vi "RANGE Gas Meters.vi"() -> ()   [LabVIEW 2016]
uses:
  Type Definitions/RANGE DAQ Data Four Meters.ctl
  Type Definitions/RANGE DAQ Data.ctl
  Drivers/Omega FMA-1600A Series Gas Flow Meter/Type Definitions/FMA1600A Gas Type.ctl
  Drivers/Omega FMA-1600A Series Gas Flow Meter/Type Definitions/FMA1600A Units String.ctl
  Type Definitions/RANGE GAS Data.ctl
  Type Definitions/RANGE Panel Data.ctl
  Type Definitions/RANGE Meter Selector 1-2.ctl
  Type Definitions/RANGE Meter Selector 3-4.ctl
  Type Definitions/RANGE Meter Selector 5-6.ctl
  Drivers/Omega FMA-1600A Series Gas Flow Meter/Type Definitions/FMA1600A Commands.ctl
  Utility/Type Definitions/UTILITY Notifier.ctl
  Utility/Custom Pallet Controls/Custom Pallet DBL.ctl
  Type Definitions/Range Meter Bank.ctl
panel:
  in  "Tab Control 2":T1(tab)
  out "Bank 3 Gas Pres":string
  out "Bank 3 Gas Temp":string
  out "Bank 3 Tot. Flow":string
  out "Bank 3 Vol Flow":string
  out "Bank 3 Mass Flow":string
  out "Bank 2 Gas Pres":string
  out "Bank 2 Gas Temp":string
  out "Bank 2 Tot. Flow":string
  out "Bank 2 Vol Flow":string
  out "Bank 2 Mass Flow":string
  out "Bank 1 Gas Pres":string
  out "Bank 1 Gas Temp":string
  out "Bank 1 Tot. Flow":string
  out "Bank 1 Vol Flow":string
  in  "Tare Meter Bank 3":bool
  in  "Change Gas Meter Bank 3":bool
  in  "Gas Type 3":T2
  in  "Tare Meter Bank 2":bool
  in  "Change Gas Meter Bank 2":bool
  in  "Gas Type 2":T2
  in  "Tare Meter Bank 1":bool
  out "Flow Rate":dbl caption="Flow Rate (BTU/hr)" format="%#_5f"
  out "DisplayChart":cluster{"Flow Rate (BTU/HR)":dbl}(graph)
  in  "HeatingValueS1":dbl=2450.0 min=2400.0 max=2600.0 step=1.0
  in  "Meter Select":T3
  out "Flow Rate 2":dbl caption="Flow Rate (BTU/hr)" format="%#_5f"
  out "DisplayChart 2":cluster{"Flow Rate (BTU/HR)":dbl}(graph)
  in  "HeatingValueS2":dbl=2450.0 min=900.0 max=2600.0 step=1.0
  in  "Meter Select 2":T4 caption="Meter Select"
  out "Flow Rate 3":dbl caption="Flow Rate (BTU/hr)" format="%#_5f"
  out "DisplayChart 3":cluster{"Flow Rate (BTU/HR)":dbl}(graph)
  in  "HeatingValueS3":dbl=2450.0 min=900.0 max=2600.0 step=1.0
  in  "Meter Select 3":T5 caption="Meter Select"
  out "Display Bank 2":T6
  out "Display Bank 3":T6
  out "ANSI Display 3":string
  in  "Start ANSI 3":bool
  out "ANSI Average (BTU/hr) 3":dbl caption="ANSI Average (BTU/hr)" format="%#_5g"
  out "ANSI Display 2":string
  in  "Start ANSI 2":bool
  out "ANSI Average (BTU/hr) 2":dbl caption="ANSI Average (BTU/hr)" format="%#_5g"
  out "ANSI Display 1":string
  in  "Start ANSI":bool
  out "ANSI Average (BTU/hr)":dbl format="%#_5g"
  in  "Change Gas Meter Bank1":bool
  in  "Gas Type":T2
  in  "Reset Totalizer Bank 1":bool
  in  "Reset Totalizer Bank 2":bool
  in  "Reset Totalizer Bank 3":bool
  out "Bank 1 Mass Flow":string
  out "Display Bank 1":T6
  out "Meter Software 1/2":string
  out "Meter Software 3/4":string
  out "Meter Software 5/6":string
  out "Bank 1 Tot. Flow":string
  out "Bank 1 Gas Pres":string
  out "Bank 1 Gas Temp":string
  out "Bank 1 Vol Flow":string
  out "Bank 1 Mass Flow":string
  out "Display S1":T7
  out "Station 1 Chart":cluster{"Flow Rate (BTU/HR)":dbl}(graph)
  out "Flow Rate S1":dbl caption="Flow Rate (BTU/hr)" format="%#_5g"
  out "ANSI Display S1":string caption="ANSI Display 1"
  in  "Start ANSI-S1":bool
  out "ANSI Average (BTU/hr)-Meter 1/2":dbl format="%#_5g"
  in  "HeatingValue Meter 1/2":dbl=2450.0 min=2400.0 max=2600.0 step=1.0
  in  "Meter Select 1/2":T3
  out "Meter 1/2":string caption="Meter"
  out "Bank 2 Mass Flow 2":string
  out "Bank 2 Vol Flow 3":string
  out "Bank 2 Gas Temp 3":string
  out "Bank 2 Gas Pres 3":string
  out "Bank 2 Tot. Flow 3":string
  out "Station 2 Chart":cluster{"Flow Rate (BTU/HR)":dbl}(graph)
  out "ANSI Display S2":string caption="ANSI Display 1"
  in  "Start ANSI-S2":bool
  out "ANSI Average (BTU/hr)-Meter 3/4":dbl format="%#_5g"
  out "Flow Rate S2":dbl caption="Flow Rate (BTU/hr)" format="%#_5g"
  out "Display S2":T7
  in  "HeatingValue Meter 3/4":dbl=2450.0 min=2400.0 max=2600.0 step=1.0
  in  "Meter Select 3/4":T4 caption="Meter Select 3-4"
  out "Meter 3/4":string caption="Meter"
  out "Bank 3 Mass Flow":string
  out "Bank 3 Vol Flow":string
  out "Bank 3 Gas Temp":string
  out "Bank 3 Gas Pres":string
  out "Bank 3 Tot. Flow":string
  out "Station 3 Chart":cluster{"Flow Rate (BTU/HR)":dbl}(graph)
  out "Flow Rate S3":dbl caption="Flow Rate (BTU/hr)" format="%#_5g"
  out "ANSI Display S3":string caption="ANSI Display 1"
  in  "Start ANSI-S3":bool
  out "ANSI Average (BTU/hr)-Meter 5/6":dbl format="%#_5g"
  out "Display S3":T7
  in  "HeatingValue Meter 5/6":dbl=2450.0 min=2400.0 max=2600.0 step=1.0
  in  "Meter Select 5/6":T5 caption="Meter Select 5-6"
  out "Meter 5/6":string caption="Meter"
  in  "Manual Commands":bool
  in  "Gas Mix Number Bank 3":string="242"
  in  "Gas Mix Number Bank 2":string="241"
  in  "Gas Mix Number Bank 1":string="240"
  in  "Custom Gas Mixture Bank 1":string="A GM TST 240 90.00 1 10.00 0"
  in  "Tab Control 3":T8(tab)
  in  "Custom Gas Mixture":string="E GM TST 240 90.00 1 10.00 0"
  in  "Custom Gas Mixture 2":string="C GM TST 240 90.00 1 10.00 0"
  in  "FMA1600A Commands":T9="*w42=31730"
  out "Raw FMA1600A Data":string
  in  "Unit ID (A-F)":string
  in  "Scan Rate (Sec)":dbl=1.0
  in  "Exit Button":bool
  out "Elapsed Time":dbl format="%<%H:%M:%S>t"
  out "File  Version":string="Parametric Stand"
  in  "Record":bool
  in  "File Path":path
  in  "Tab Control":enum32{"Debug Data", "Page 2", "Page 3"}(tab)
  out "Error Out":errorcluster
  in  "Error In":errorcluster
  out "All Meter Data":T10={"Meter 1"={"Meter Size"=0.0, "DAQ Output (Voltage)"=0.0, "Reference (Voltage)"=0.0, "Meter Present"=FALSE, "Meter Visa"="COM3", "Gas Type"="", "SLPM Error @ Zero"=0.0, "Gas Mix Number"="", "Set STP Register"=FALSE, "Measurement Units"={"Abs. Pressure"="", "Gauge/Diff. Press."="", "Barometric Press."="", "Temperature"="", "Volume"="", "Mass"="", "Setpoint"="", "Valve Drive"="", "Totalizer"="", "Tot. Timer"="", "Tot. Avg. Flow"="", "Tot. Peak Flow"="", "Software Version"=""}}, "Meter 2"={"Meter Size"=0.0, "DAQ Output (Voltage)"=0.0, "Reference (Voltage)"=0.0, "Meter Present"=FALSE, "Meter Visa"="COM4", "Gas Type"="", "SLPM Error @ Zero"=0.0, "Gas Mix Number"="", "Set STP Register"=FALSE, "Measurement Units"={"Abs. Pressure"="", "Gauge/Diff. Press."="", "Barometric Press."="", "Temperature"="", "Volume"="", "Mass"="", "Setpoint"="", "Valve Drive"="", "Totalizer"="", "Tot. Timer"="", "Tot. Avg. Flow"="", "Tot. Peak Flow"="", "Software Version"=""}}, "Meter 3"={"Meter Size"=0.0, "DAQ Output (Voltage)"=0.0, "Reference (Voltage)"=0.0, "Meter Present"=FALSE, "Meter Visa"="COM5", "Gas Type"="", "SLPM Error @ Zero"=0.0, "Gas Mix Number"="", "Set STP Register"=FALSE, "Measurement Units"={"Abs. Pressure"="", "Gauge/Diff. Press."="", "Barometric Press."="", "Temperature"="", "Volume"="", "Mass"="", "Setpoint"="", "Valve Drive"="", "Totalizer"="", "Tot. Timer"="", "Tot. Avg. Flow"="", "Tot. Peak Flow"="", "Software Version"=""}}, "Meter 4"={"Meter Size"=0.0, "DAQ Output (Voltage)"=0.0, "Reference (Voltage)"=0.0, "Meter Present"=FALSE, "Meter Visa"="COM6", "Gas Type"="", "SLPM Error @ Zero"=0.0, "Gas Mix Number"="", "Set STP Register"=FALSE, "Measurement Units"={"Abs. Pressure"="", "Gauge/Diff. Press."="", "Barometric Press."="", "Temperature"="", "Volume"="", "Mass"="", "Setpoint"="", "Valve Drive"="", "Totalizer"="", "Tot. Timer"="", "Tot. Avg. Flow"="", "Tot. Peak Flow"="", "Software Version"=""}}, "Meter 5"={"Meter Size"=0.0, "DAQ Output (Voltage)"=0.0, "Reference (Voltage)"=0.0, "Meter Present"=FALSE, "Meter Visa"="COM7", "Gas Type"="", "SLPM Error @ Zero"=0.0, "Gas Mix Number"="", "Set STP Register"=FALSE, "Measurement Units"={"Abs. Pressure"="", "Gauge/Diff. Press."="", "Barometric Press."="", "Temperature"="", "Volume"="", "Mass"="", "Setpoint"="", "Valve Drive"="", "Totalizer"="", "Tot. Timer"="", "Tot. Avg. Flow"="", "Tot. Peak Flow"="", "Software Version"=""}}, "Meter 6"={"Meter Size"=0.0, "DAQ Output (Voltage)"=0.0, "Reference (Voltage)"=0.0, "Meter Present"=FALSE, "Meter Visa"="COM8", "Gas Type"="", "SLPM Error @ Zero"=0.0, "Gas Mix Number"="", "Set STP Register"=FALSE, "Measurement Units"={"Abs. Pressure"="", "Gauge/Diff. Press."="", "Barometric Press."="", "Temperature"="", "Volume"="", "Mass"="", "Setpoint"="", "Valve Drive"="", "Totalizer"="", "Tot. Timer"="", "Tot. Avg. Flow"="", "Tot. Peak Flow"="", "Software Version"=""}}, "Meter Bank 1"={"Flow Rate (BTU/HR)"=0.0, "ANSI Placeholder Array"=[], "15 Sec Avg Array"=[], "30 Sec Avg Array "=[], "ANSI Average (BTU/HR)"=0.0, "Panel Data"={"Meter Type (Gas)"="", "Heating Value (BTU/ft³)"=0.0, "Ft³ / Hr (SCFH)"=0.0, "15 Second Average (BTU/HR)"=0.0, "30 Second Average (BTU/HR)"=0.0, "Mass Flow"=0.0, "Vol. Flow"=0.0, "Gas Temperature"=0.0, "Gas Pressure"=0.0, "Tot.Flow"=0.0}, "Start ANSI"=FALSE, "ANSI Start Time"=0.0, "Restart ANSI"=FALSE, "Meter ID"=""}, "Meter Bank 2"={"Flow Rate (BTU/HR)"=0.0, "ANSI Placeholder Array"=[], "15 Sec Avg Array"=[], "30 Sec Avg Array "=[], "ANSI Average (BTU/HR)"=0.0, "Panel Data"={"Meter Type (Gas)"="", "Heating Value (BTU/ft³)"=0.0, "Ft³ / Hr (SCFH)"=0.0, "15 Second Average (BTU/HR)"=0.0, "30 Second Average (BTU/HR)"=0.0, "Mass Flow"=0.0, "Vol. Flow"=0.0, "Gas Temperature"=0.0, "Gas Pressure"=0.0, "Tot.Flow"=0.0}, "Start ANSI"=FALSE, "ANSI Start Time"=0.0, "Restart ANSI"=FALSE, "Meter ID"=""}, "Meter Bank 3"={"Flow Rate (BTU/HR)"=0.0, "ANSI Placeholder Array"=[], "15 Sec Avg Array"=[], "30 Sec Avg Array "=[], "ANSI Average (BTU/HR)"=0.0, "Panel Data"={"Meter Type (Gas)"="", "Heating Value (BTU/ft³)"=0.0, "Ft³ / Hr (SCFH)"=0.0, "15 Second Average (BTU/HR)"=0.0, "30 Second Average (BTU/HR)"=0.0, "Mass Flow"=0.0, "Vol. Flow"=0.0, "Gas Temperature"=0.0, "Gas Pressure"=0.0, "Tot.Flow"=0.0}, "Start ANSI"=FALSE, "ANSI Start Time"=0.0, "Restart ANSI"=FALSE, "Meter ID"=""}, "Threshold Voltage (NI DAQ)"=0.2, "Use RS232 Data Collection"=FALSE, "Use Auto Switching"=FALSE}
  out "Main Loop Rate":dbl format="%0.2f"
  out "Tot.Flow (SLPM Liters) Bank 1":dbl
  out "Tot.Flow (SLPM Liters) Bank 2":dbl
  out "Tot.Flow (SLPM Liters) Bank 3":dbl
  out "Average Updates":T10={"Meter 1"={"Meter Size"=0.0, "DAQ Output (Voltage)"=0.0, "Reference (Voltage)"=0.0, "Meter Present"=FALSE, "Meter Visa"="COM3", "Gas Type"="", "SLPM Error @ Zero"=0.0, "Gas Mix Number"="", "Set STP Register"=FALSE, "Measurement Units"={"Abs. Pressure"="", "Gauge/Diff. Press."="", "Barometric Press."="", "Temperature"="", "Volume"="", "Mass"="", "Setpoint"="", "Valve Drive"="", "Totalizer"="", "Tot. Timer"="", "Tot. Avg. Flow"="", "Tot. Peak Flow"="", "Software Version"=""}}, "Meter 2"={"Meter Size"=0.0, "DAQ Output (Voltage)"=0.0, "Reference (Voltage)"=0.0, "Meter Present"=FALSE, "Meter Visa"="COM3", "Gas Type"="", "SLPM Error @ Zero"=0.0, "Gas Mix Number"="", "Set STP Register"=FALSE, "Measurement Units"={"Abs. Pressure"="", "Gauge/Diff. Press."="", "Barometric Press."="", "Temperature"="", "Volume"="", "Mass"="", "Setpoint"="", "Valve Drive"="", "Totalizer"="", "Tot. Timer"="", "Tot. Avg. Flow"="", "Tot. Peak Flow"="", "Software Version"=""}}, "Meter 3"={"Meter Size"=0.0, "DAQ Output (Voltage)"=0.0, "Reference (Voltage)"=0.0, "Meter Present"=FALSE, "Meter Visa"="COM3", "Gas Type"="", "SLPM Error @ Zero"=0.0, "Gas Mix Number"="", "Set STP Register"=FALSE, "Measurement Units"={"Abs. Pressure"="", "Gauge/Diff. Press."="", "Barometric Press."="", "Temperature"="", "Volume"="", "Mass"="", "Setpoint"="", "Valve Drive"="", "Totalizer"="", "Tot. Timer"="", "Tot. Avg. Flow"="", "Tot. Peak Flow"="", "Software Version"=""}}, "Meter 4"={"Meter Size"=0.0, "DAQ Output (Voltage)"=0.0, "Reference (Voltage)"=0.0, "Meter Present"=FALSE, "Meter Visa"="COM3", "Gas Type"="", "SLPM Error @ Zero"=0.0, "Gas Mix Number"="", "Set STP Register"=FALSE, "Measurement Units"={"Abs. Pressure"="", "Gauge/Diff. Press."="", "Barometric Press."="", "Temperature"="", "Volume"="", "Mass"="", "Setpoint"="", "Valve Drive"="", "Totalizer"="", "Tot. Timer"="", "Tot. Avg. Flow"="", "Tot. Peak Flow"="", "Software Version"=""}}, "Meter 5"={"Meter Size"=0.0, "DAQ Output (Voltage)"=0.0, "Reference (Voltage)"=0.0, "Meter Present"=FALSE, "Meter Visa"="COM3", "Gas Type"="", "SLPM Error @ Zero"=0.0, "Gas Mix Number"="", "Set STP Register"=FALSE, "Measurement Units"={"Abs. Pressure"="", "Gauge/Diff. Press."="", "Barometric Press."="", "Temperature"="", "Volume"="", "Mass"="", "Setpoint"="", "Valve Drive"="", "Totalizer"="", "Tot. Timer"="", "Tot. Avg. Flow"="", "Tot. Peak Flow"="", "Software Version"=""}}, "Meter 6"={"Meter Size"=0.0, "DAQ Output (Voltage)"=0.0, "Reference (Voltage)"=0.0, "Meter Present"=FALSE, "Meter Visa"="COM3", "Gas Type"="", "SLPM Error @ Zero"=0.0, "Gas Mix Number"="", "Set STP Register"=FALSE, "Measurement Units"={"Abs. Pressure"="", "Gauge/Diff. Press."="", "Barometric Press."="", "Temperature"="", "Volume"="", "Mass"="", "Setpoint"="", "Valve Drive"="", "Totalizer"="", "Tot. Timer"="", "Tot. Avg. Flow"="", "Tot. Peak Flow"="", "Software Version"=""}}, "Meter Bank 1"={"Flow Rate (BTU/HR)"=0.0, "ANSI Placeholder Array"=[], "15 Sec Avg Array"=[], "30 Sec Avg Array "=[], "ANSI Average (BTU/HR)"=0.0, "Panel Data"={"Meter Type (Gas)"="", "Heating Value (BTU/ft³)"=0.0, "Ft³ / Hr (SCFH)"=0.0, "15 Second Average (BTU/HR)"=0.0, "30 Second Average (BTU/HR)"=0.0, "Mass Flow"=0.0, "Vol. Flow"=0.0, "Gas Temperature"=0.0, "Gas Pressure"=0.0, "Tot.Flow"=0.0}, "Start ANSI"=FALSE, "ANSI Start Time"=0.0, "Restart ANSI"=FALSE, "Meter ID"=""}, "Meter Bank 2"={"Flow Rate (BTU/HR)"=0.0, "ANSI Placeholder Array"=[], "15 Sec Avg Array"=[], "30 Sec Avg Array "=[], "ANSI Average (BTU/HR)"=0.0, "Panel Data"={"Meter Type (Gas)"="", "Heating Value (BTU/ft³)"=0.0, "Ft³ / Hr (SCFH)"=0.0, "15 Second Average (BTU/HR)"=0.0, "30 Second Average (BTU/HR)"=0.0, "Mass Flow"=0.0, "Vol. Flow"=0.0, "Gas Temperature"=0.0, "Gas Pressure"=0.0, "Tot.Flow"=0.0}, "Start ANSI"=FALSE, "ANSI Start Time"=0.0, "Restart ANSI"=FALSE, "Meter ID"=""}, "Meter Bank 3"={"Flow Rate (BTU/HR)"=0.0, "ANSI Placeholder Array"=[], "15 Sec Avg Array"=[], "30 Sec Avg Array "=[], "ANSI Average (BTU/HR)"=0.0, "Panel Data"={"Meter Type (Gas)"="", "Heating Value (BTU/ft³)"=0.0, "Ft³ / Hr (SCFH)"=0.0, "15 Second Average (BTU/HR)"=0.0, "30 Second Average (BTU/HR)"=0.0, "Mass Flow"=0.0, "Vol. Flow"=0.0, "Gas Temperature"=0.0, "Gas Pressure"=0.0, "Tot.Flow"=0.0}, "Start ANSI"=FALSE, "ANSI Start Time"=0.0, "Restart ANSI"=FALSE, "Meter ID"=""}, "Threshold Voltage (NI DAQ)"=0.2, "Use RS232 Data Collection"=FALSE, "Use Auto Switching"=FALSE}
  in  "Min to Sec Convert (Total Flow)":dbl=60.0 format="%#_13g"
  in  "Rate Threshold (V)":dbl=0.02
  out "ANSI 1":bool
  out "ANSI 2":bool
  out "ANSI 3":bool
  out "Gas Total Loop":i32
  out "ANSI Loop":i32
  out "Main Control Loop":i32
  out "Debug Array":string[](array[string])
  in  "Debug":bool
  out "Save Loop":i32
  out "Event Loop":i32
  out "Num Record":dbl
  # "Meter 1 & 2"
  # "Meter 3 & 4"
  # "Meter 5 & 6"
  # "Heating Value (BTU/ft³)"
  # "Heating Value (BTU/ft³)"
  # "Heating Value (BTU/ft³)"
  # "Custom Commands\nAuthorized ONLY"
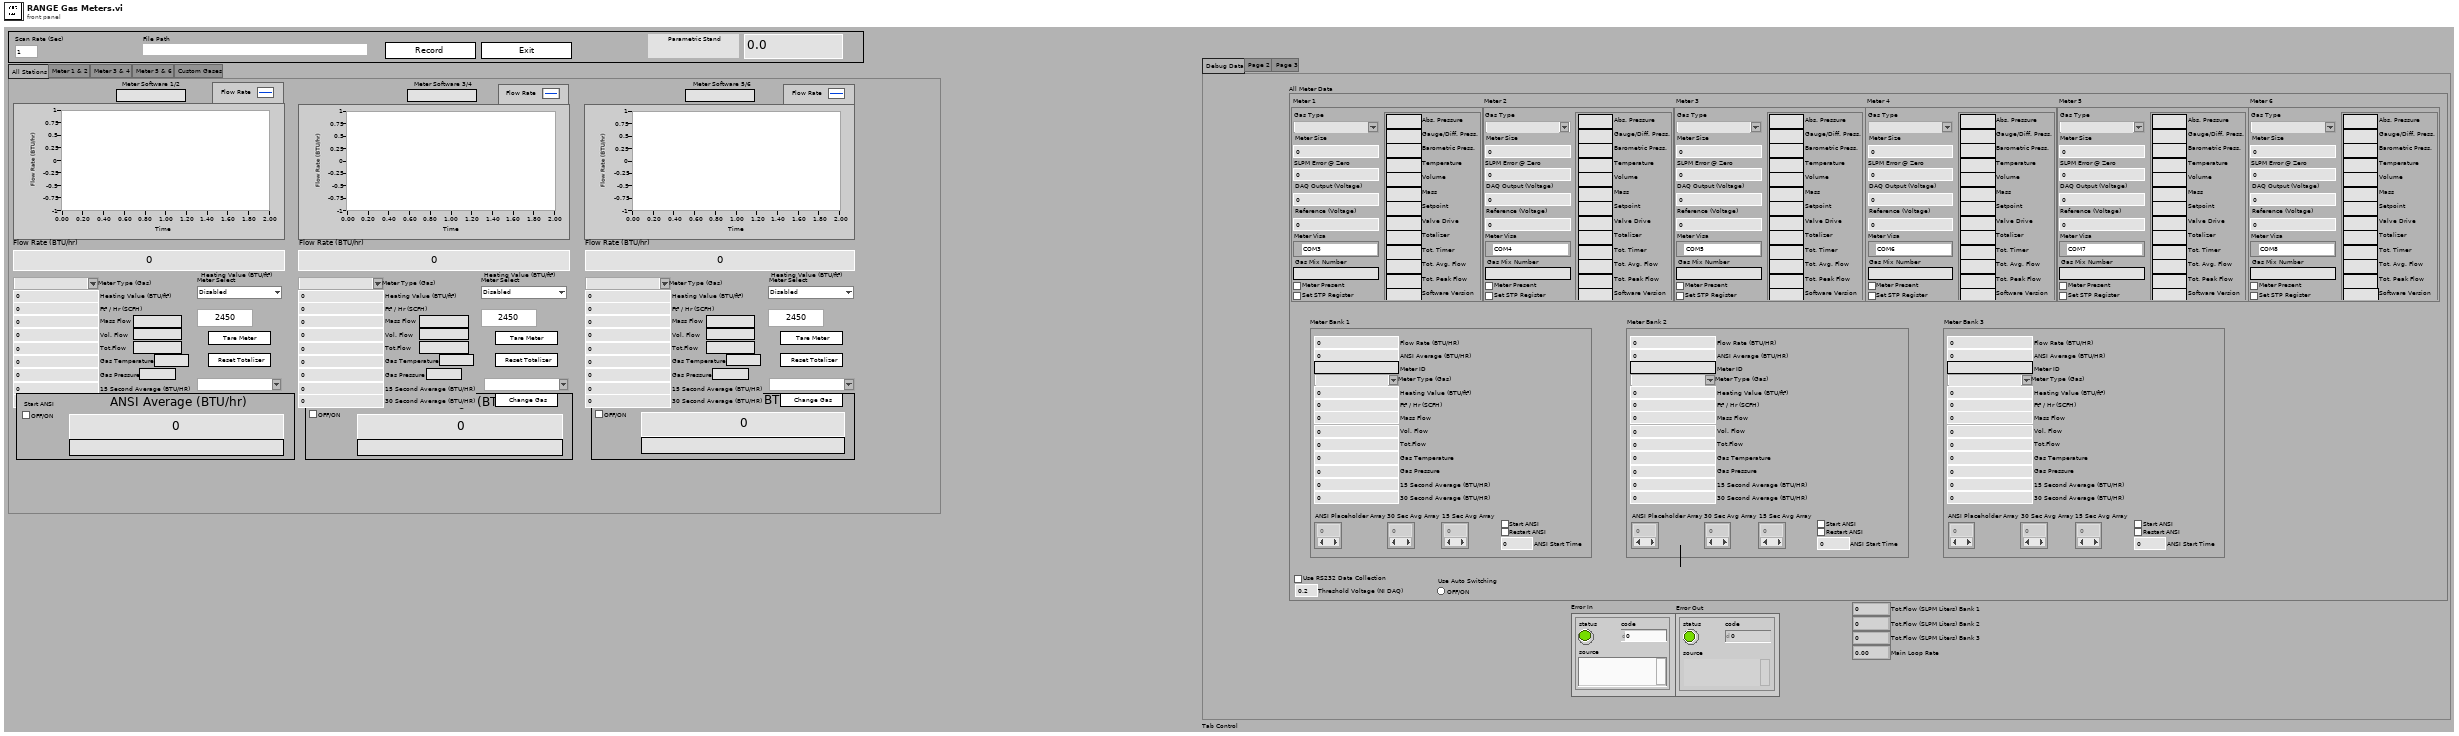
[diagram p1: front panel]
types:
  T1 = enum32{"All Stations", "Meter 1 & 2", "Meter 3 & 4", "Meter 5 & 6", "Custom Gases"}
  T2 = typedef "FMA1600A Gas Type.ctl" = string
  T3 = typedef "RANGE Meter Selector 1-2.ctl" = enum16{"Disabled", "Meter 1", "Meter 2", "Auto"}
  T4 = typedef "RANGE Meter Selector 3-4.ctl" = enum16{"Disabled", "Meter 3", "Meter 4", "Auto"}
  T5 = typedef "RANGE Meter Selector 5-6.ctl" = enum16{"Disabled", "Meter 5", "Meter 6", "Auto"}
  T6 = typedef "RANGE Panel Data.ctl" = cluster{"Meter Type (Gas)":T2, "Heating Value (BTU/ft³)":dbl, "Ft³ / Hr (SCFH)":dbl, "15 Second Average (BTU/HR)":dbl, "30 Second Average (BTU/HR)":dbl, "Mass Flow":dbl, "Vol. Flow":dbl, "Gas Temperature":dbl, "Gas Pressure":dbl, "Tot.Flow":dbl}
  T7 = cluster{"Meter Type (Gas)":T2, "Heating Value (BTU/ft³)":dbl, "Ft³ / Hr (SCFH)":dbl, "15 Second Average (BTU/HR)":dbl, "30 Second Average (BTU/HR)":dbl, "Mass Flow":dbl, "Vol. Flow":dbl, "Gas Temperature":dbl, "Gas Pressure":dbl, "Tot.Flow":dbl}
  T8 = enum32{"General Gases", "Pure Non-Corrosice Gases", "Pure Corrosive", "Refrigerants", "Welding Gases", "BioReactor Gases", "Breathing Gases", "Fuel Gases", "Laser Gases", "Create Gas Mixture"}
  T9 = typedef "FMA1600A Commands.ctl" = string
  T10 = typedef "RANGE DAQ Data Four Meters.ctl" = cluster{"Meter 1":T11, "Meter 2":T11, "Meter 3":T11, "Meter 4":T11, "Meter 5":T11, "Meter 6":T11, "Meter Bank 1":T13, "Meter Bank 2":T13, "Meter Bank 3":T13, "Threshold Voltage (NI DAQ)":dbl, "Use RS232 Data Collection":bool, "Use Auto Switching":bool}
  T11 = typedef "RANGE DAQ Data.ctl" = cluster{"Meter Size":dbl, "DAQ Output (Voltage)":dbl, "Reference (Voltage)":dbl, "Meter Present":bool, "Meter Visa":refnum<visa-resource-name>, "Gas Type":T2, "SLPM Error @ Zero":dbl, "Gas Mix Number":string, "Set STP Register":bool, "Measurement Units":T12}
  T12 = typedef "FMA1600A Units String.ctl" = cluster{"Abs. Pressure":string, "Gauge/Diff. Press.":string, "Barometric Press.":string, "Temperature":string, "Volume":string, "Mass":string, "Setpoint":string, "Valve Drive":string, "Totalizer":string, "Tot. Timer":string, "Tot. Avg. Flow":string, "Tot. Peak Flow":string, "Software Version":string}
  T13 = typedef "RANGE GAS Data.ctl" = cluster{"Flow Rate (BTU/HR)":dbl, "ANSI Placeholder Array":dbl[], "15 Sec Avg Array":dbl[], "30 Sec Avg Array ":dbl[], "ANSI Average (BTU/HR)":dbl, "Panel Data":T6, "Start ANSI":bool, "ANSI Start Time":dbl, "Restart ANSI":bool, "Meter ID":string}
  T14 = typedef "UTILITY Notifier.ctl" = enum16{"Set", "Read", "Release Ref"}
  T15 = enum8{"Enabled", "Disabled", "Disabled and Grayed Out"}
  T16 = typedef "FileVersionInformation.ctl" = cluster{"FileVersion":string, "ProductName":string, "InternalName":string, "CompanyName":string, "LegalCopyright":string, "FileDescription":string}
  T17 = enum32{"invalid app kind", "Development System", "Run Time System", "Student Edition", "Embedded LabVIEW", "Evaluation", "Custom"}
  T18 = enum32{"Invalid", "Standard", "Closed", "Hidden", "Minimized", "Maximized"}
  T19 = typedef "Range Meter Bank.ctl" = enum16{"Meter Bank 1", "Meter Bank 2", "Meter Bank 3"}
  T20 = cluster{"Core":cluster{"Current VI Reference":refnum<vi>, "Close Panel on Exit?":bool}, "Bank 1 Counter":i32, "Bank 2 Counter":i32, "Bank 3 Counter":i32, "Meter Data":T10, "File Path":path, "Start Data Save":bool, "Elapsed Time DAQ":dbl}
  T21 = cluster{"Current VI Reference":refnum<vi>, "Close Panel on Exit?":bool}
  T22 = typedef "Custom Pallet DBL.ctl" = dbl
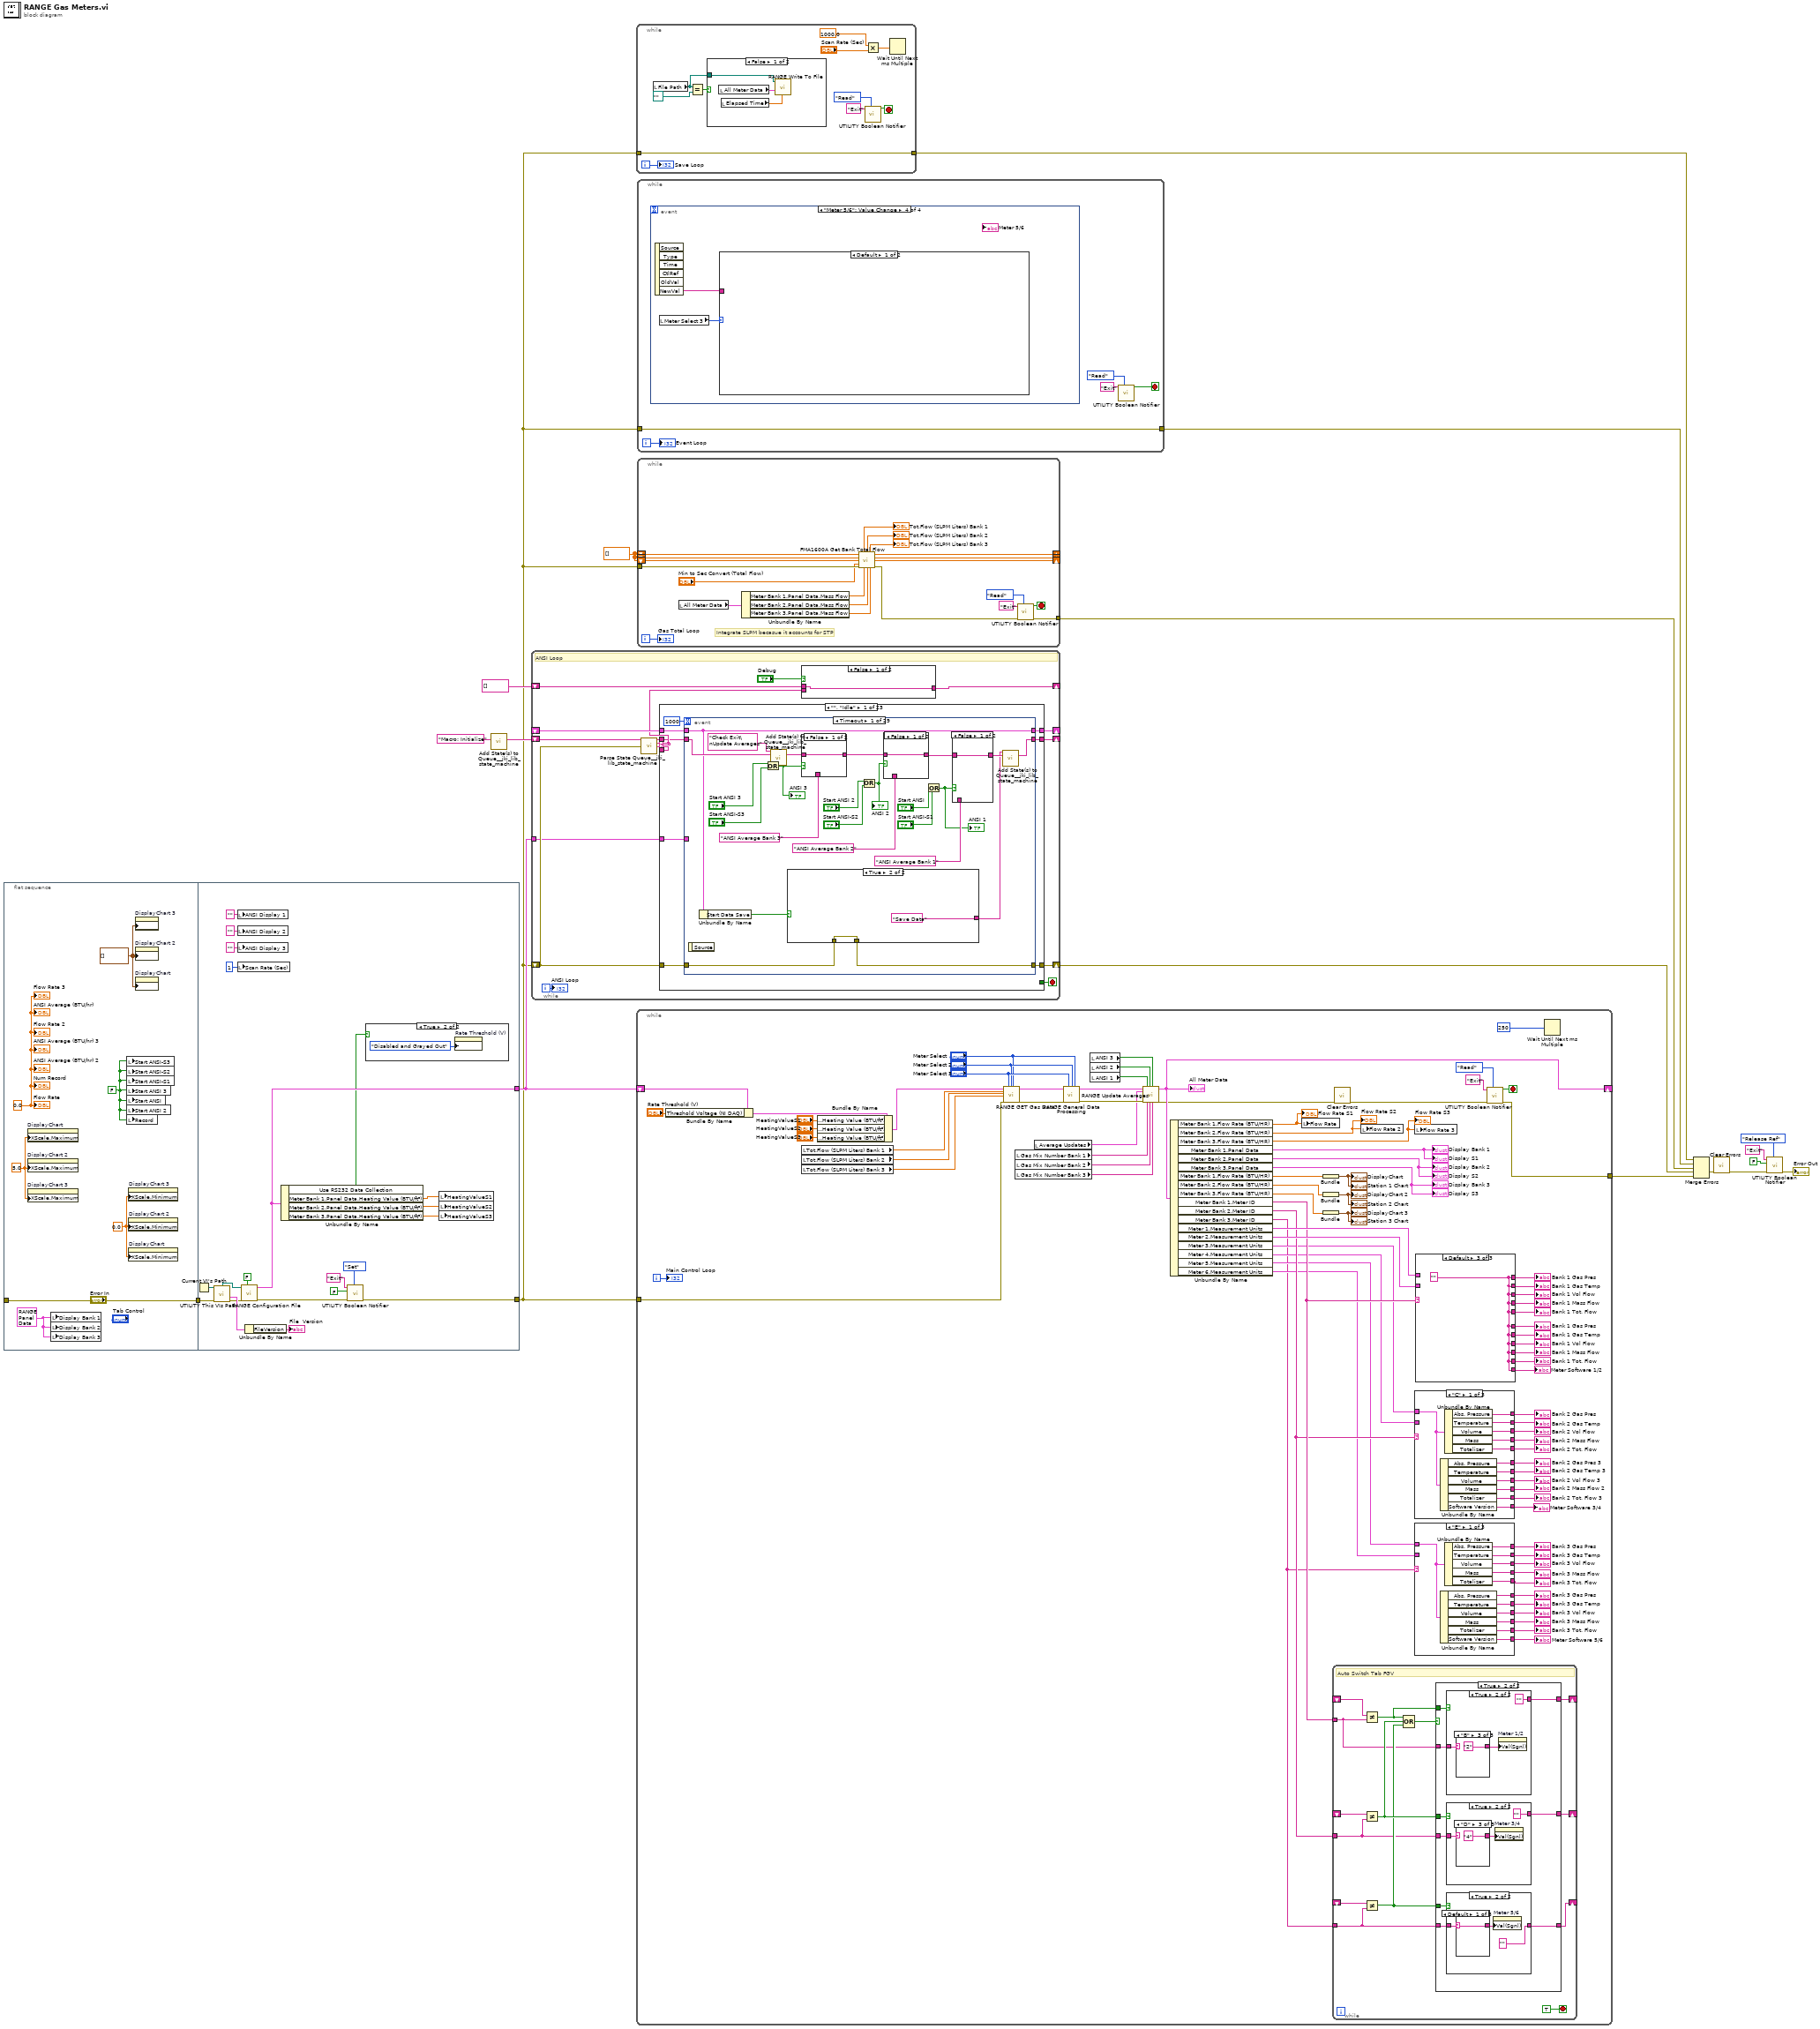
[diagram p0: block diagram]
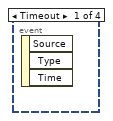
[diagram p3: hidden frame]
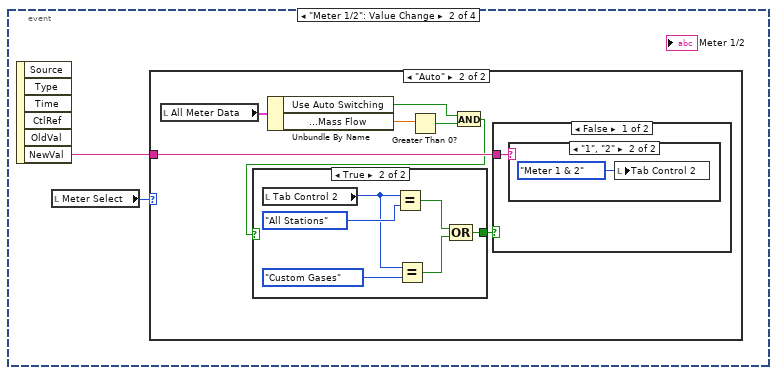
[diagram p4: hidden frame]
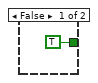
[diagram p6: hidden frame]
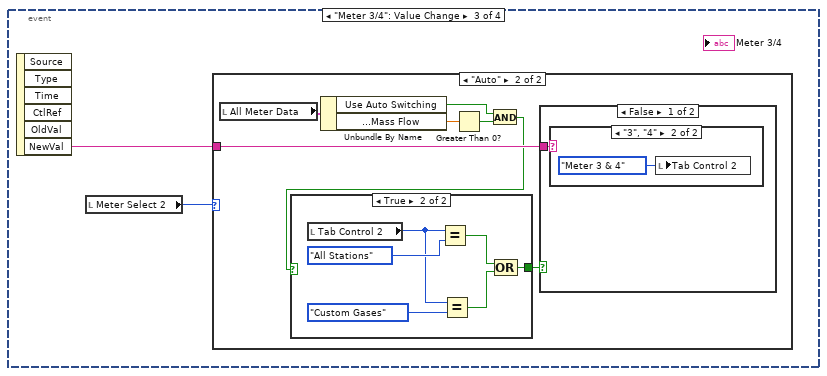
[diagram p9: hidden frame]
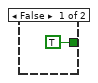
[diagram p11: hidden frame]
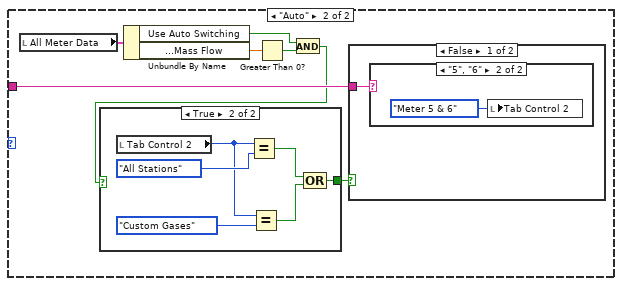
[diagram p14: hidden frame]
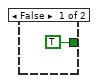
[diagram p15: hidden frame]
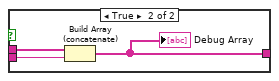
[diagram p18: hidden frame]
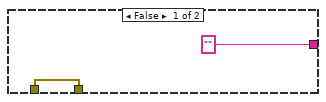
[diagram p19: hidden frame]
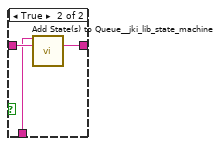
[diagram p20: hidden frame]
diagram:
  w13 = dbl[] []
  n1 = flat-sequence {
    tunnel: "Error In" -> [w21]
    tunnel: [w21] -> w18
    tunnel: w18 -> [w44]
    tunnel: [w28] -> w3
    tunnel: [w41] -> w12
    frame #0 {
      w22 = 5.0
      w23 = 0.0
      w20 = FALSE
      w24 = T6 {"Meter Type (Gas)"="", "Heating Value (BTU/ft³)"=0.0, "Ft³ / Hr (SCFH)"=0.0, "15 Second Average (BTU/HR)"=0.0, "30 Second Average (BTU/HR)"=0.0, "Mass Flow"=0.0, "Vol. Flow"=0.0, "Gas Temperature"=0.0, "Gas Pressure"=0.0, "Tot.Flow"=0.0} ("Display Bank 1")
      w25 = 0.0
      w26 = cluster{"[0]":dbl}[] []
      n2 = property on="DisplayChart" class="WFChart (strict)"("XScale.Maximum"=w22) -> ()  [unwired: 2 in, 2 out]
      n3 = property on="DisplayChart 2" class="WFChart (strict)"("XScale.Maximum"=w22) -> ()  [unwired: 2 in, 2 out]
      n4 = property on="DisplayChart 3" class="WFChart (strict)"("XScale.Maximum"=w22) -> ()  [unwired: 2 in, 2 out]
      n5 = local write "Display Bank 1"(w24) -> ()
      n6 = local write "Display Bank 2"(w24) -> ()
      n7 = local write "Display Bank 3"(w24) -> ()
      n8 = local write "Start ANSI-S3"(w20) -> ()
      n9 = local write "Start ANSI-S2"(w20) -> ()
      n10 = local write "Start ANSI-S1"(w20) -> ()
      n11 = local write "Start ANSI 3"(w20) -> ()
      n12 = local write "Start ANSI"(w20) -> ()
      n13 = local write "Start ANSI 2"(w20) -> ()
      n14 = local write "Record"(w20) -> ()
      n15 = property on="DisplayChart 3" class="WFChart (strict)"("XScale.Minimum"=w23) -> ()  [unwired: 2 in, 2 out]
      n16 = property on="DisplayChart 2" class="WFChart (strict)"("XScale.Minimum"=w23) -> ()  [unwired: 2 in, 2 out]
      n17 = property on="DisplayChart" class="WFChart (strict)"("XScale.Minimum"=w23) -> ()  [unwired: 2 in, 2 out]
      n18 = property on="DisplayChart 3" class="WFChart (strict)"("History Data"=w26) -> ()  [unwired: 2 in, 2 out]
      n19 = property on="DisplayChart 2" class="WFChart (strict)"("History Data"=w26) -> ()  [unwired: 2 in, 2 out]
      n20 = property on="DisplayChart" class="WFChart (strict)"("History Data"=w26) -> ()  [unwired: 2 in, 2 out]
      "Num Record" <- w25
      "ANSI Average (BTU/hr)" <- w25
      "Flow Rate" <- w25
      "Flow Rate 2" <- w25
      "ANSI Average (BTU/hr) 2" <- w25
      "Flow Rate 3" <- w25
      "ANSI Average (BTU/hr) 3" <- w25
    }
    frame #1 {
      n21 = Current VI's Path() -> (path=w47:path)
      n22 = call "UTILITY This VIs Path.vi"("path"=w47, "error in (no error)"=w44) -> ("Folder Path"=w39:path, "FileVersionInfo Out"=w46:T16, "error out"=w43:errorcluster)  [unwired: 7 in, 4 out]
      n23 = local write "ANSI Display 1"("" ("ANSI Display 1")) -> ()
      n24 = local write "ANSI Display 2"("" ("ANSI Display 2")) -> ()
      n25 = local write "ANSI Display 3"("" ("ANSI Display 3")) -> ()
      n26 = local write "Scan Rate (Sec)"(1 ("Scan Rate (Sec)")) -> ()
      n27 = call "RANGE Configuration File.vi"("Debug"=FALSE, "Error In"=w43, "Gas Lab Config File"=w39) -> ("Error Out"=w29:errorcluster, "Meter Data"=w41:T10)  [unwired: 7 in]
      n28 = Unbundle By Name(w46) -> ("FileVersion"=→"File  Version":string)
      n29 = Unbundle By Name(w41) -> ("Use RS232 Data Collection"=w40:bool, "Meter Bank 1.Panel Data.Heating Value (BTU/ft³)"=w35:dbl, "Meter Bank 2.Panel Data.Heating Value (BTU/ft³)"=w34:dbl, "Meter Bank 3.Panel Data.Heating Value (BTU/ft³)"=w33:dbl)
      n30 = call "UTILITY Boolean Notifier.vi"("Status"=UTILITY_Notifier."Set", "error in (no error)"=w29, "Set Status"=FALSE, "name (unnamed)"="Exit") -> ("error out"=w28:errorcluster)  [unwired: 6 in, 1 out]
      n31 = case shown="True" w40 {
        frame False {
          n32 = property on="Rate Threshold (V)" class="DigNum (strict)"("DisabledEnum"=T15."Enabled" ("Disabled")) -> ()  [unwired: 2 in, 2 out]
        }
        frame True {
          n33 = property on="Rate Threshold (V)" class="DigNum (strict)"("DisabledEnum"=T15."Disabled and Grayed Out" ("Disabled")) -> ()  [unwired: 2 in, 2 out]
        }
      }
      n34 = local write "HeatingValueS1"(w35) -> ()
      n35 = local write "HeatingValueS2"(w34) -> ()
      n36 = local write "HeatingValueS3"(w33) -> ()
    }
  }
  n37 = call <vilib>:"Add State(s) to Queue__jki_lib_state_machine.vi"("State(s) in (\"\")"="Macro: Initialize") -> ("States Out"=w17:string)  [unwired: 14 in]
  n38 = while "ANSI Loop" {
    shift-right: [w58] -> _
    shift-left: _ -> [w57]
    shift-right: [w61] -> w14
    shift-left: w3 -> [w56]
    shift-right: [w60] -> _
    shift-left: w17 -> [w62]
    tunnel: w12 -> [w55]
    shift-right: [w52] -> _
    shift-left: string[] [] -> [w53]
    i -> [w54]
    stop <- w59 stop-if-true
    # "ANSI Loop"
    n39 = call <vilib>:"Parse State Queue__jki_lib_state_machine.vi"("State Queue"=w62, "Error In (no error)"=w56) -> ("Remaining States"=w64:string, "Current State"=w51:string, "Arguments"=w63:string)  [unwired: 11 in]
    n40 = case shown="\"\", \"Idle\"" w51 {
      selector: w51 -> [_ _ w401 _ _ _ _ _ _ _ _ _ _ _ _ _ _ _ _ _ _ _ _]
      tunnel: w64 -> [w76 w400 w405 w423 w429 w436 w444 w456 w462 w466 w470 w476 w487 w513 w518 w528 w532 w555 w569 w584 w599 w604 w612]
      tunnel: w63 -> [_ _ _ _ _ _ _ _ _ _ _ w471 w481 _ _ _ _ _ _ _ _ _ _]
      tunnel: w57 -> [w74 w397 w403 w414 w426 w434 w441 _ w457 w463 w468 w474 w483 w510 w515 w525 w529 w539 w566 w575 w591 w602 w610]
      tunnel: [w73 w398 w407 w420 errorcluster {"status"=FALSE, "code"=0, "source"=""} ("error out") w430 w442 w453 w458 w464 w467 w472 w484 w511 w516 w526 w530 w534 w562 w576 w590 w601 w609] -> w61
      tunnel: w56 -> [w72 w398 w406 w420 w425 w431 w442 w453 w459 w464 w467 w473 w485 w511 w516 w526 w530 w541 w563 w577 w593 w601 w609]
      tunnel: [w75 w399 w404 w422 w428 w435 w443 w455 w461 w465 w469 w475 w486 w512 w517 w527 w531 w554 w568 w583 w598 w603 w611] -> w60
      tunnel: [_ _ _ _ _ w432 _ _ _ _ _ _ _ _ _ _ _ _ _ _ _ _ _] -> w59
      tunnel: [w71 w397 w403 w421 w426 w434 w441 w454 w457 w463 w468 w474 w483 w510 w515 w525 w529 w538 w565 w579 w592 w602 w610] -> w58
      tunnel: w55 -> [w70 _ _ _ _ _ _ w448 _ _ _ _ _ _ _ _ _ _ _ _ _ _ _]
      frame "", "Idle" {
        n41 = event shown="[0] Timeout" {
          selector: _ -> [_ _ _ _ _ _ _ _ _ _ _ _ _ _ _ _ _ _ _ _ _ _ _ _ _ _ _ _ _]
          dyn-events: _ -> [_ _ _ _ _ _ _ _ _ _ _ _ _ _ _ _ _ _ _ _ _ _ _ _ _ _ _ _ _]
          timeout: 1000 -> [_ _ _ _ _ _ _ _ _ _ _ _ _ _ _ _ _ _ _ _ _ _ _ _ _ _ _ _ _]
          tunnel: w76 -> [w100 w122 w128 w134 w135 w147 w169 w171 w181 w191 w203 w223 w271 w275 w279 w281 w286 w291 w295 w298 w302 w306 w311 w315 w326 w349 w372 w388 w394]
          tunnel: [w85 w122 w128 w134 w135 w147 w169 w171 w181 w191 w203 w223 w271 w275 w279 w281 w286 w291 w295 w298 w302 w306 w311 w315 w326 w349 w372 w387 w393] -> w75
          tunnel: w74 -> [w84 w120 w126 w132 w136 w148 w170 w172 w182 w192 w205 w224 w272 w276 w280 w282 w287 w292 w296 w299 w303 w307 w312 w316 w327 w350 w373 w389 w395]
          tunnel: [w80 w121 w127 w133 w137 w149 w159 w173 w183 w194 w206 w220 w269 w273 w278 w283 w285 w290 w294 w300 w304 w308 w310 w314 w323 w346 w369 w390 w391] -> w73
          tunnel: w72 -> [w81 w121 w127 w133 w138 w150 w161 w174 w184 w195 w207 w221 w269 w273 w278 w283 w285 w290 w294 w300 w304 w308 w310 w314 w324 w348 w371 w390 w391]
          tunnel: [w84 w119 w125 w131 w136 w148 w170 w172 w182 w192 w204 w224 w272 w276 w280 w282 w287 w292 w296 w299 w303 w307 w312 w316 w327 w350 w373 w389 w395] -> w71
          tunnel: w70 -> [_ _ _ _ w139 w151 w160 w175 w185 w193 _ w219 _ _ _ _ _ _ _ _ _ _ _ _ w317 w340 w363 _ _]
          event Timeout {
            n42 = event-data() -> ()  [unwired: 1 in, 1 out]
            n43 = Unbundle By Name(w84) -> ("Start Data Save"=w82:bool)
            n44 = Or(x="Start ANSI 3", y="Start ANSI-S3") -> (x .or. y?=w79:bool)
            "ANSI 3" <- w79
            n45 = call <vilib>:"Add State(s) to Queue__jki_lib_state_machine.vi"("State(s) in Front (\"\")"="Check Exit\nUpdate Averages" ("State(s) in Front (\"\")"), "State(s) in (\"\")"=w100) -> ("States Out"=w98:string)  [unwired: 13 in]
            n46 = case shown="True" w82 {
              tunnel: ["" ("State(s) in Front (\"\")") "Save Data" ("State(s) in Front (\"\")")] -> w83
              tunnel: w81 -> [w101 w103]
              tunnel: [w101 w103] -> w80
              frame False {
              }
              frame True {
              }
            }
            n47 = case shown="False" w79 {
              tunnel: w98 -> [w113 w116]
              tunnel: [w113 w115] -> w97
              tunnel: "ANSI Average Bank 3" ("State(s) in Front (\"\")") -> [_ w114]
              frame False {
              }
              frame True {
                n48 = call <vilib>:"Add State(s) to Queue__jki_lib_state_machine.vi"("State(s) in Front (\"\")"=w114, "State(s) in (\"\")"=w116) -> ("States Out"=w115:string)  [unwired: 13 in]
              }
            }
            n49 = Or(x="Start ANSI 2", y="Start ANSI-S2") -> (x .or. y?=w77:bool)
            "ANSI 2" <- w77
            n50 = case shown="False" w77 {
              tunnel: w97 -> [w109 w112]
              tunnel: [w109 w111] -> w96
              tunnel: "ANSI Average Bank 2" ("State(s) in Front (\"\")") -> [_ w110]
              frame False {
              }
              frame True {
                n51 = call <vilib>:"Add State(s) to Queue__jki_lib_state_machine.vi"("State(s) in Front (\"\")"=w110, "State(s) in (\"\")"=w112) -> ("States Out"=w111:string)  [unwired: 13 in]
              }
            }
            n52 = Or(x="Start ANSI", y="Start ANSI-S1") -> (x .or. y?=w78:bool)
            "ANSI 1" <- w78
            n53 = case shown="False" w78 {
              tunnel: w96 -> [w105 w108]
              tunnel: [w105 w107] -> w86
              tunnel: "ANSI Average Bank 1" ("State(s) in Front (\"\")") -> [_ w106]
              frame False {
              }
              frame True {
                n54 = call <vilib>:"Add State(s) to Queue__jki_lib_state_machine.vi"("State(s) in Front (\"\")"=w106, "State(s) in (\"\")"=w108) -> ("States Out"=w107:string)  [unwired: 13 in]
              }
            }
            n55 = call <vilib>:"Add State(s) to Queue__jki_lib_state_machine.vi"("State(s) in Front (\"\")"=w83, "State(s) in (\"\")"=w86) -> ("States Out"=w85:string)  [unwired: 13 in]
          }
          event "Start ANSI": Value Change {
            n56 = event-data() -> ()  [unwired: 1 in, 6 out]
            n57 = local write "ANSI Display 1"("" ("ANSI Display 1")) -> ()
            n58 = Bundle By Name(cluster=w120, "Bank 1 Counter"=0) -> (w119:T20)
          }
          event "Start ANSI 2": Value Change {
            n59 = event-data() -> ()  [unwired: 1 in, 6 out]
            n60 = Bundle By Name(cluster=w126, "Bank 2 Counter"=0) -> (w125:T20)
            n61 = local write "ANSI Display 2"("" ("ANSI Display 2")) -> ()
          }
          event "Start ANSI 3": Value Change {
            n62 = event-data() -> ()  [unwired: 1 in, 6 out]
            n63 = local write "ANSI Display 3"("" ("ANSI Display 3")) -> ()
            n64 = Bundle By Name(cluster=w132, "Bank 3 Counter"=0) -> (w131:T20)
          }
          event "Change Gas Meter Bank1": Value Change {
            n65 = event-data() -> ()  [unwired: 1 in, 6 out]
            n66 = local read "Meter Select"() -> (w144:T3)
            n67 = call "RANGE Meter Bank Select.vi"("Error In"=w138, "Meter Data"=w139, "Meter Select"=w144) -> ("Error Out"=w142:errorcluster, "Unit ID"=w143:string, "VISA Refnum out"=w141:refnum<visa-resource-name>)  [unwired: 6 in]
            n68 = call "FMA1600A Create Custom Gas Mixture.vi"("Gas Mix Number"="Gas Mix Number Bank 1", "Gas Type"="Gas Type", "Error In"=w142, "Custom Gas Mixture"="Custom Gas Mixture Bank 1", "Unit ID"=w143, "VISA Refnum in"=w141) -> ("Error Out"=w137:errorcluster)  [unwired: 5 in]
          }
          event "Change Gas Meter Bank 2": Value Change {
            n69 = event-data() -> ()  [unwired: 1 in, 6 out]
            n70 = local read "Meter Select 2"() -> (w156:T4)
            n71 = call "RANGE Meter Bank Select 2.vi"("Error In"=w150, "Meter Data"=w151, "Meter Select 2"=w156) -> ("Error Out"=w158:errorcluster, "Unit ID"=w155:string, "VISA Refnum out"=w157:refnum<visa-resource-name>)  [unwired: 6 in]
            n72 = call "FMA1600A Create Custom Gas Mixture.vi"("Gas Mix Number"="Gas Mix Number Bank 2", "Gas Type"="Gas Type 2", "Error In"=w158, "Custom Gas Mixture"="Custom Gas Mixture 2", "Unit ID"=w155, "VISA Refnum in"=w157) -> ("Error Out"=w149:errorcluster)  [unwired: 5 in]
          }
          event "Change Gas Meter Bank 3": Value Change {
            n73 = event-data() -> ()  [unwired: 1 in, 6 out]
            n74 = local read "Meter Select 3"() -> (w168:T5)
            n75 = call "RANGE Meter Bank Select 3.vi"("Error In"=w161, "Meter Data"=w160, "Meter Select Bank 3"=w168) -> ("Error Out"=w167:errorcluster, "Unit ID"=w164:string, "VISA Refnum out"=w165:refnum<visa-resource-name>)  [unwired: 6 in]
            n76 = call "FMA1600A Create Custom Gas Mixture.vi"("Gas Mix Number"="Gas Mix Number Bank 3", "Gas Type"="Gas Type 3", "Error In"=w167, "Custom Gas Mixture"="Custom Gas Mixture", "Unit ID"=w164, "VISA Refnum in"=w165) -> ("Error Out"=w159:errorcluster)  [unwired: 5 in]
          }
          event "Tare Meter Bank 1": Value Change {
            n77 = event-data() -> ()  [unwired: 1 in, 6 out]
            n78 = local read "Meter Select"() -> (w180:T3)
            n79 = call "RANGE Meter Bank Select.vi"("Error In"=w174, "Meter Data"=w175, "Meter Select"=w180) -> ("Error Out"=w176:errorcluster, "Unit ID"=w179:string, "VISA Refnum out"=w177:refnum<visa-resource-name>)  [unwired: 6 in]
            n80 = call "FMA1600A Send Receive.vi"("Unit ID"=w179, "error in (no error)"=w176, "FMA1600A Commands"=T9 "$$V", "VISA Refnum in"=w177) -> ("error out"=w173:errorcluster)  [unwired: 5 in, 2 out]
          }
          event "Tare Meter Bank 2": Value Change {
            n81 = event-data() -> ()  [unwired: 1 in, 6 out]
            n82 = local read "Meter Select 2"() -> (w187:T4)
            n83 = call "RANGE Meter Bank Select 2.vi"("Error In"=w184, "Meter Data"=w185, "Meter Select 2"=w187) -> ("Error Out"=w186:errorcluster, "Unit ID"=w190:string, "VISA Refnum out"=w188:refnum<visa-resource-name>)  [unwired: 6 in]
            n84 = call "FMA1600A Send Receive.vi"("Unit ID"=w190, "error in (no error)"=w186, "FMA1600A Commands"=T9 "$$V", "VISA Refnum in"=w188) -> ("error out"=w183:errorcluster)  [unwired: 5 in, 2 out]
          }
          event "Tare Meter Bank 3": Value Change {
            n85 = event-data() -> ()  [unwired: 1 in, 6 out]
            n86 = local read "Meter Select 3"() -> (w197:T5)
            n87 = call "RANGE Meter Bank Select 3.vi"("Error In"=w195, "Meter Data"=w193, "Meter Select Bank 3"=w197) -> ("Error Out"=w196:errorcluster, "Unit ID"=w200:string, "VISA Refnum out"=w198:refnum<visa-resource-name>)  [unwired: 6 in]
            n88 = call "FMA1600A Send Receive.vi"("Unit ID"=w200, "error in (no error)"=w196, "FMA1600A Commands"=T9 "$$V", "VISA Refnum in"=w198) -> ("error out"=w194:errorcluster)  [unwired: 5 in, 2 out]
          }
          event "Record": Value Change {
            n89 = event-data() -> ("NewVal"=w202:bool)  [unwired: 1 in, 5 out]
            n90 = case shown="True" w202 {
              tunnel: w207 -> [w209 w216]
              tunnel: [w209 w215] -> w206
              tunnel: [path "" ("Path") w214] -> w201
              frame False {
              }
              frame True {
                n91 = local read "Meter 3/4"() -> (w210:string)
                n92 = local read "Meter 1/2"() -> (w211:string)
                n93 = local read "All Meter Data"() -> (w213:T10)
                n94 = local read "Meter 5/6"() -> (w212:string)
                n95 = call "RANGE Create File.vi"("Meter 3/4"=w210, "Meter 5/6"=w212, "Meter 1/2"=w211, "Error In"=w216, "All Meter Data"=w213) -> ("Error Out"=w215:errorcluster, "Path"=w214:path)  [unwired: 5 in]
              }
            }
            n96 = local write "File Path"(w201) -> ()
            n97 = Bundle By Name(cluster=w205, "Start Data Save"=w202, "File Path"=w201) -> (w204:T20)
          }
          event "Manual Commands": Value Change {
            n98 = event-data() -> ()  [unwired: 1 in, 6 out]
            n99 = case shown="\"A\"" "Unit ID (A-F)" {
              tunnel: "FMA1600A Commands" -> [_ w232 w239 w242 w251 w256 w263]
              tunnel: w221 -> [w226 w229 w238 w243 w248 w260 w267]
              tunnel: [w226 w228 w237 w244 w253 w259 w266] -> w220
              tunnel: "Unit ID (A-F)" -> [_ w231 w234 w241 w250 w255 w264]
              tunnel: w219 -> [_ w233 w240 w247 w254 w261 w268]
              tunnel: ["" ("Raw FMA1600A Data") w227 w235 w245 w252 w258 w265] -> w217
              frame Default {
              }
              frame "A" {
                n100 = Unbundle By Name(w233) -> ("Meter 1.Meter Visa"=w230:refnum<visa-resource-name>)
                n101 = call "FMA1600A General Send Receive.vi"("error in (no error)"=w229, "Unit ID in"=w231, "FMA1600A Commands"=w232, "VISA Refnum in"=w230) -> ("error out"=w228:errorcluster, "Data Stream"=w227:string)  [unwired: 4 in, 2 out]
              }
              frame "B" {
                n102 = Unbundle By Name(w240) -> ("Meter 2.Meter Visa"=w236:refnum<visa-resource-name>)
                n103 = call "FMA1600A General Send Receive.vi"("error in (no error)"=w238, "Unit ID in"=w234, "FMA1600A Commands"=w239, "VISA Refnum in"=w236) -> ("error out"=w237:errorcluster, "Data Stream"=w235:string)  [unwired: 4 in, 2 out]
              }
              frame "C" {
                n104 = Unbundle By Name(w247) -> ("Meter 3.Meter Visa"=w246:refnum<visa-resource-name>)
                n105 = call "FMA1600A General Send Receive.vi"("error in (no error)"=w243, "Unit ID in"=w241, "FMA1600A Commands"=w242, "VISA Refnum in"=w246) -> ("error out"=w244:errorcluster, "Data Stream"=w245:string)  [unwired: 4 in, 2 out]
              }
              frame "D" {
                n106 = Unbundle By Name(w254) -> ("Meter 4.Meter Visa"=w249:refnum<visa-resource-name>)
                n107 = call "FMA1600A General Send Receive.vi"("error in (no error)"=w248, "Unit ID in"=w250, "FMA1600A Commands"=w251, "VISA Refnum in"=w249) -> ("error out"=w253:errorcluster, "Data Stream"=w252:string)  [unwired: 4 in, 2 out]
              }
              frame "E" {
                n108 = Unbundle By Name(w261) -> ("Meter 5.Meter Visa"=w257:refnum<visa-resource-name>)
                n109 = call "FMA1600A General Send Receive.vi"("error in (no error)"=w260, "Unit ID in"=w255, "FMA1600A Commands"=w256, "VISA Refnum in"=w257) -> ("error out"=w259:errorcluster, "Data Stream"=w258:string)  [unwired: 4 in, 2 out]
              }
              frame "F" {
                n110 = Unbundle By Name(w268) -> ("Meter 6.Meter Visa"=w262:refnum<visa-resource-name>)
                n111 = call "FMA1600A General Send Receive.vi"("error in (no error)"=w267, "Unit ID in"=w264, "FMA1600A Commands"=w263, "VISA Refnum in"=w262) -> ("error out"=w266:errorcluster, "Data Stream"=w265:string)  [unwired: 4 in, 2 out]
              }
            }
            "Raw FMA1600A Data" <- w217
          }
          event "HeatingValueS1": Value Change {
            n112 = event-data() -> ()  [unwired: 1 in, 6 out]
            n113 = local read "HeatingValueS1"() -> (w270:dbl)
            n114 = local write "HeatingValue Meter 1/2"(w270) -> ()
          }
          event "HeatingValueS2": Value Change {
            n115 = event-data() -> ()  [unwired: 1 in, 6 out]
            n116 = local read "HeatingValueS2"() -> (w274:dbl)
            n117 = local write "HeatingValue Meter 3/4"(w274) -> ()
          }
          event "HeatingValueS3": Value Change {
            n118 = event-data() -> ()  [unwired: 1 in, 6 out]
            n119 = local read "HeatingValueS3"() -> (w277:dbl)
            n120 = local write "HeatingValue Meter 5/6"(w277) -> ()
          }
          event "HeatingValue Meter 1/2": Value Change {
            n121 = event-data() -> ()  [unwired: 1 in, 6 out]
            n122 = local read "HeatingValue Meter 1/2"() -> (w284:dbl)
            n123 = local write "HeatingValueS1"(w284) -> ()
          }
          event "HeatingValue Meter 3/4": Value Change {
            n124 = event-data() -> ()  [unwired: 1 in, 6 out]
            n125 = local read "HeatingValue Meter 3/4"() -> (w288:dbl)
            n126 = local write "HeatingValueS2"(w288) -> ()
          }
          event "HeatingValue Meter 5/6": Value Change {
            n127 = event-data() -> ()  [unwired: 1 in, 6 out]
            n128 = local read "HeatingValue Meter 5/6"() -> (w289:dbl)
            n129 = local write "HeatingValueS3"(w289) -> ()
          }
          event Value Change {
            n130 = event-data() -> ()  [unwired: 1 in, 6 out]
            n131 = local read "Meter Select"() -> (w293:T3)
            n132 = local write "Meter Select 1/2"(w293) -> ()
          }
          event Value Change {
            n133 = event-data() -> ()  [unwired: 1 in, 6 out]
            n134 = local read "Meter Select 2"() -> (w297:T4)
            n135 = local write "Meter Select 3/4"(w297) -> ()
          }
          event Value Change {
            n136 = event-data() -> ()  [unwired: 1 in, 6 out]
            n137 = local read "Meter Select 3"() -> (w301:T5)
            n138 = local write "Meter Select 5/6"(w301) -> ()
          }
          event Value Change {
            n139 = event-data() -> ()  [unwired: 1 in, 6 out]
            n140 = local write "Meter Select"("Meter Select 1/2") -> ()
          }
          event Value Change {
            n141 = event-data() -> ()  [unwired: 1 in, 6 out]
            n142 = local write "Meter Select 2"("Meter Select 3/4") -> ()
          }
          event Value Change {
            n143 = event-data() -> ()  [unwired: 1 in, 6 out]
            n144 = local write "Meter Select 3"("Meter Select 5/6") -> ()
          }
          event "Reset Totalizer Bank 1": Value Change {
            n145 = event-data() -> ()  [unwired: 1 in, 6 out]
            n146 = local read "Meter Select"() -> (w319:T3)
            n147 = call "RANGE Meter Bank Select.vi"("Error In"=w324, "Meter Data"=w317, "Meter Select"=w319) -> ("Error Out"=w325:errorcluster, "Unit ID"=w318:string, "VISA Refnum out"=w322:refnum<visa-resource-name>)  [unwired: 6 in]
            n148 = Equal?(x=refnum<visa-resource-name> refnum, y=w322) -> (x = y?=w320:bool)
            n149 = case shown="False" w320 {
              tunnel: w325 -> [w331 w339]
              tunnel: [w330 w339] -> w323
              tunnel: w322 -> [w329 _]
              tunnel: w318 -> [w328 _]
              frame False {
                n150 = for {
                  N: 5 -> [_]
                  tunnel: w328 -> [w334]
                  shift-right: [w335] -> w330
                  shift-left: w331 -> [w338]
                  shift-right: [w336] -> _
                  shift-left: w329 -> [w337]
                  # "If you have a totalizer model. It \nrequires a different command to clear"
                  n151 = call "FMA1600A Send Receive.vi"("Unit ID"=w334, "error in (no error)"=w338, "FMA1600A Commands"=T9 "$$T", "VISA Refnum in"=w337) -> ("error out"=w335:errorcluster, "VISA Refnum out"=w336:refnum<visa-resource-name>)  [unwired: 5 in, 1 out]
                }
              }
              frame True {
              }
            }
          }
          event "Reset Totalizer Bank 2": Value Change {
            n152 = event-data() -> ()  [unwired: 1 in, 6 out]
            n153 = local read "Meter Select 2"() -> (w342:T4)
            n154 = call "RANGE Meter Bank Select 2.vi"("Error In"=w348, "Meter Data"=w340, "Meter Select 2"=w342) -> ("Error Out"=w347:errorcluster, "Unit ID"=w341:string, "VISA Refnum out"=w345:refnum<visa-resource-name>)  [unwired: 6 in]
            n155 = Equal?(x=refnum<visa-resource-name> refnum, y=w345) -> (x = y?=w343:bool)
            n156 = case shown="False" w343 {
              tunnel: w347 -> [w354 w362]
              tunnel: [w353 w362] -> w346
              tunnel: w345 -> [w352 _]
              tunnel: w341 -> [w351 _]
              frame False {
                n157 = for {
                  N: 5 -> [_]
                  tunnel: w351 -> [w357]
                  shift-right: [w358] -> w353
                  shift-left: w354 -> [w361]
                  shift-right: [w359] -> _
                  shift-left: w352 -> [w360]
                  # "If you have a totalizer model. It \nrequires a different command to clear"
                  n158 = call "FMA1600A Send Receive.vi"("Unit ID"=w357, "error in (no error)"=w361, "FMA1600A Commands"=T9 "$$T", "VISA Refnum in"=w360) -> ("error out"=w358:errorcluster, "VISA Refnum out"=w359:refnum<visa-resource-name>)  [unwired: 5 in, 1 out]
                }
              }
              frame True {
              }
            }
          }
          event "Reset Totalizer Bank 3": Value Change {
            n159 = event-data() -> ()  [unwired: 1 in, 6 out]
            n160 = local read "Meter Select 3"() -> (w365:T5)
            n161 = call "RANGE Meter Bank Select 3.vi"("Error In"=w371, "Meter Data"=w363, "Meter Select Bank 3"=w365) -> ("Error Out"=w370:errorcluster, "Unit ID"=w364:string, "VISA Refnum out"=w368:refnum<visa-resource-name>)  [unwired: 6 in]
            n162 = Equal?(x=refnum<visa-resource-name> refnum, y=w368) -> (x = y?=w366:bool)
            n163 = case shown="False" w366 {
              tunnel: w370 -> [w377 w385]
              tunnel: w368 -> [w376 _]
              tunnel: [w375 w385] -> w369
              tunnel: w364 -> [w374 _]
              frame False {
                n164 = for {
                  N: 5 -> [_]
                  tunnel: w374 -> [w380]
                  shift-right: [w381] -> w375
                  shift-left: w377 -> [w384]
                  shift-right: [w382] -> _
                  shift-left: w376 -> [w383]
                  # "If you have a totalizer model. It \nrequires a different command to clear"
                  n165 = call "FMA1600A Send Receive.vi"("Unit ID"=w380, "error in (no error)"=w384, "FMA1600A Commands"=T9 "$$T", "VISA Refnum in"=w383) -> ("error out"=w381:errorcluster, "VISA Refnum out"=w382:refnum<visa-resource-name>)  [unwired: 5 in, 1 out]
                }
              }
              frame True {
              }
            }
          }
          event "Exit Button": Value Change {
            n166 = event-data() -> ()  [unwired: 1 in, 6 out]
            n167 = call <vilib>:"Add State(s) to Queue__jki_lib_state_machine.vi"("State(s) in Front (\"\")"="Macro: Exit" ("State(s) in Front (\"\")"), "State(s) in (\"\")"=w388) -> ("States Out"=w387:string)  [unwired: 13 in]
          }
          event Panel Close? {
            n168 = event-data() -> ()  [unwired: 1 in, 4 out]
            n169 = call <vilib>:"Add State(s) to Queue__jki_lib_state_machine.vi"("State(s) in Front (\"\")"="Macro: Exit" ("State(s) in Front (\"\")"), "State(s) in (\"\")"=w394) -> ("States Out"=w393:string)  [unwired: 13 in]
            n170 = event-data("Discard?"=TRUE) -> ()  [unwired: 1 in, 1 out]
          }
        }
      }
      frame "---------- Core ----------" {
        # "Do not put any code in this frame.\n(it is a separator no-op)"
        n171 = call <vilib>:"Add State(s) to Queue__jki_lib_state_machine.vi"("State(s) in (\"\")"=w400) -> ("States Out"=w399:string)  [unwired: 14 in]
      }
      frame Default {
        w410 = 42 items=["No error", "Argument error", "Memory is full", "Out of zone", "End of file", "File already open", "Generic file I/O error", "File not found", "File permission error", "Disk is full", "Duplicate path", "Too many files open", "System feature not enabled", "Resource file not found", "Cannot add resource", "Resource not found", "Image not found", "Image memory error", "Pen does not exist", "Config type invalid", "Config token not found", "Config parse error", "Config memory error", "Bad external code format", "Bad external code offset", "External code not present", "Null window", "Destroy window error", "Null menu", "Print aborted", "Bad print record", "Print driver error", "Windows error during printing", "Memory error during printing", "Print dialog error", "Generic print error", "Invalid device refnum", "Device not found", "Device parameter error", "Device unit error", "Cannot open device", "Device call aborted", "Generic error", "Cancelled by user", "Object ID too low", "Object ID too high", "Object not in heap", "Unknown heap", "Unknown object (invalid DefProc)", "Unknown object (DefProc not in table)", "Message out of range", "Invalid (null) method", "Unknown message", "Manager call not supported", "Bad address", "Network operation in progress", "Network operation timed out", "Connection is busy", "Network attribute not supported", "Network error", "Address in use", "System out of memory", "Connection aborted", "Connection refused", "Not connected", "Already connected", "Connection closed", "Initialization error (interapplication manager)", "Bad occurrence", "Wait on unbound occurrence handler", "Occurrence queue overflow", "Datalog type conflict", "Unused", "Unrecognized type (interapplication manager)", "Memory corrupt", "Failed to make temporary DLL", "Old CIN version", "Drag socket not found", "Failed to load drop-object", "Failed to register OLE object", "Failed to release OLE object", "Format specifier type mismatch", "Unknown format specifier", "Too few format specifiers", "Too many format specifiers", "Scan failed", "Newer CIN version", "Error converting to variant", "Runtime menu error", "Password tampered", "Variant attribute not found", "Incompatible variant data type", "Event data is not available", "Event Store is not present", "Occurrence is not found", "Event Queue is not created", "Event info is not available", "Refnum passed is NULL", "Error retrieving Class GUID", "Error retrieving CoClass GUID", "Error retrieving TypeLib GUID.", "Bad built application magic bytes.", "Specific driver is different from the specific driver associated with the Logical Name.", "There is no session opened to the class driver.", "Max Error", "MAX - Error with config objects", "MAX - Error loading configuration", "MAX - Group not supported"]
        # "Current State"
        # "Do not delete, rename, or modify this frame.\n(this is used to capture unhandled states and typos)"
        # "Handle mistyped state name (developer tool)"
        n172 = Format Into String(format string="Software Exception: Unhandled State \"%s\"." ("message"), error in=w406, w401) -> (resulting string=w409:string, error out=w408:errorcluster)  [unwired: 1 in]
        n173 = call <vilib>:"Error Cluster From Error Code.vi"("show call chain? (False)"=TRUE, "error in (no error)"=w408, "error message (\"\")"=w409, "error code (0)"=w410) -> ("error out"=w407:errorcluster)  [unwired: 5 in]
        n174 = call <vilib>:"Add State(s) to Queue__jki_lib_state_machine.vi"("State(s) in (\"\")"=w405) -> ("States Out"=w404:string)  [unwired: 14 in]
      }
      frame "Initialize Core Data" {
        # "Do not delete, rename, or modify this frame.\n(this is used to determine panel behavior on exit)"
        # "originally closed?"
        # "exe?"
        # "If panel starts closed or is an EXE, then close it when we exit"
        n175 = property class="VI"() -> ("Front Panel.Open"=w419:bool)  [unwired: 2 in, 2 out]
        n176 = property class="App"() -> ("App.Kind"=w418:T17)  [unwired: 2 in, 2 out]
        n177 = control-ref of="Current VI Reference"() -> (w412:refnum<vi>)
        n178 = Not(x=w419) -> (.not. x?=w416:bool)
        n179 = Equal?(x=w418, y=T17."Run Time System" ("Application:Kind")) -> (x = y?=w415:bool)
        n180 = Or(x=w416, y=w415) -> (x .or. y?=w413:bool)
        n181 = Bundle By Name(cluster=w414, "Core.Current VI Reference"=w412, "Core.Close Panel on Exit?"=w413) -> (w421:T20)
        n182 = call <vilib>:"Add State(s) to Queue__jki_lib_state_machine.vi"("State(s) in (\"\")"=w423) -> ("States Out"=w422:string)  [unwired: 14 in]
      }
      frame "Error Handler" {
        # "Unhandled Error -- Display it"
        # "Handle any errors here.\nYou can also output any states to clean-up after errors occur"
        # "Clear error"
        n183 = call <vilib>:"General Error Handler.vi"("error in (no error)"=w425) -> ()  [unwired: 10 in, 5 out]
        n184 = call <vilib>:"Add State(s) to Queue__jki_lib_state_machine.vi"("State(s) in Front (\"\")"="/* Post Error States", "State(s) in (\"\")"=w429) -> ("States Out"=w428:string)  [unwired: 13 in]
      }
      frame "Exit" {
        w432 = TRUE
        # "Do not put any code in this frame.\n(No errors that occur here will be handled.)"
        n185 = for {
          N: 5 -> [_]
          tunnel: w432 -> [w438]
          shift-right: [w437] -> w430
          shift-left: w431 -> [w437]
          n186 = call "UTILITY Boolean Notifier.vi"("Status"=UTILITY_Notifier."Set", "Set Status"=w438, "name (unnamed)"="Exit") -> ()  [unwired: 7 in, 2 out]
        }
        n187 = call <vilib>:"Add State(s) to Queue__jki_lib_state_machine.vi"("State(s) in (\"\")"=w436) -> ("States Out"=w435:string)  [unwired: 14 in]
      }
      frame "---------- Data ----------" {
        # "Do not put any code in this frame.\n(It is a separator no-op. You can make a copy of this frame to create a new Data frame)"
        n188 = call <vilib>:"Add State(s) to Queue__jki_lib_state_machine.vi"("State(s) in (\"\")"=w444) -> ("States Out"=w443:string)  [unwired: 14 in]
      }
      frame "Data: Initialize" {
        w445 = 0.0  # Elapsed Time DAQ
        w447 = FALSE  # Start Data Save
        w449 = 0  # Bank 3 Counter
        w450 = 0  # Bank 2 Counter
        w451 = 0  # Bank 1 Counter
        w452 = T21 {"Current VI Reference"=refnum, "Close Panel on Exit?"=FALSE}  # Core
        # "These transfer data to the main heating value control"
        # "Initialize the shift-register data, here.\n(data names are defined by what you wire into the bundle function)"
        n189 = Bundle("Core"=w452, "Bank 1 Counter"=w451, "Bank 2 Counter"=w450, "Bank 3 Counter"=w449, "Meter Data"=w448, "File Path"="File Path", "Start Data Save"=w447, "Elapsed Time DAQ"=w445) -> (w454:T20)  [unwired: 1 in]
        n190 = call <vilib>:"Add State(s) to Queue__jki_lib_state_machine.vi"("State(s) in (\"\")"=w456) -> ("States Out"=w455:string)  [unwired: 14 in]
      }
      frame "Data: Cleanup" {
        # "Cleanup any data and references, here.\n(this is called automatically, by the Macro: Exit)"
        n191 = Unbundle By Name(w457) -> ("Core.Current VI Reference"=w460:refnum<vi>)
        n192 = Close Reference(reference=w460, error in (no error)=w459) -> (error out=w458:errorcluster)
        n193 = call <vilib>:"Add State(s) to Queue__jki_lib_state_machine.vi"("State(s) in (\"\")"=w462) -> ("States Out"=w461:string)  [unwired: 14 in]
      }
      frame "---------- UI ----------" {
        # "Do not put any code in this frame.\n(It is a separator no-op. You can make a copy of this frame to create a new UI frame)"
        n194 = call <vilib>:"Add State(s) to Queue__jki_lib_state_machine.vi"("State(s) in (\"\")"=w466) -> ("States Out"=w465:string)  [unwired: 14 in]
      }
      frame "UI: Initialize" {
        # "Initialize the User Interface, here.\n(this is called automatically, by the Macro: Init)"
        n195 = call <vilib>:"Add State(s) to Queue__jki_lib_state_machine.vi"("State(s) in (\"\")"=w470) -> ("States Out"=w469:string)  [unwired: 14 in]
      }
      frame "UI: Cursor Set" {
        # "Argument"
        # "Set and Unset Cursor Busy.\n(Usage: \"UI: Cursor Set >> Busy|Idle\")"
        n196 = case shown="\"Idle\", Default" w471 {
          tunnel: w473 -> [w478 w480]
          tunnel: [w477 w479] -> w472
          frame "Idle", Default {
            n197 = call <vilib>:"Unset Busy.vi"("error in (no error)"=w478) -> ("error out"=w477:errorcluster)  [unwired: 10 in]
          }
          frame "Busy" {
            n198 = call <vilib>:"Set Busy.vi"("error in (no error)"=w480) -> ("error out"=w479:errorcluster)  [unwired: 9 in, 1 out]
          }
        }
        n199 = call <vilib>:"Add State(s) to Queue__jki_lib_state_machine.vi"("State(s) in (\"\")"=w476) -> ("States Out"=w475:string)  [unwired: 14 in]
      }
      frame "UI: Front Panel State" {
        # "Argument"
        # "Set Front Panel Open or Closed\n(Usage: \"UI: Front Panel State >> Open|Close\")"
        n200 = Unbundle By Name(w483) -> ("Core.Current VI Reference"=w482:refnum<vi>)
        n201 = case shown="\"Open\", Default" w481 {
          tunnel: w485 -> [w491 w504]
          tunnel: [w493 w505] -> w484
          tunnel: w482 -> [w492 w502]
          frame "Open", Default {
            n202 = property class="VI"(reference=w492, error in=w491) -> (reference out=w489:refnum<vi>, error out=w490:errorcluster, "Front Panel.Open"=w488:bool)
            n203 = case shown="True" w488 {
              tunnel: [w496 w499] -> w493
              tunnel: w490 -> [w495 w499]
              tunnel: w489 -> [w494 _]
              frame False {
                n204 = invoke class="VI" method="FP.Open"(reference=w494, error in=w495, "Activate"=TRUE, "State"=T18."Standard") -> (error out=w496:errorcluster)  [unwired: 1 in, 4 out]
              }
              frame True {
              }
            }
          }
          frame "Close" {
            n205 = property class="VI"(reference=w502, error in=w504) -> (reference out=w501:refnum<vi>, error out=w503:errorcluster, "Front Panel.Open"=w500:bool)
            n206 = case shown="True" w500 {
              tunnel: [w506 w509] -> w505
              tunnel: w503 -> [w506 w508]
              tunnel: w501 -> [_ w507]
              frame False {
              }
              frame True {
                n207 = invoke class="VI" method="FP.Close"(reference=w507, error in=w508) -> (error out=w509:errorcluster)  [unwired: 1 in, 2 out]
              }
            }
          }
        }
        n208 = call <vilib>:"Add State(s) to Queue__jki_lib_state_machine.vi"("State(s) in (\"\")"=w487) -> ("States Out"=w486:string)  [unwired: 14 in]
      }
      frame "---------- Macro ----------" {
        # "Do not put any code in this frame.\n(It is a separator no-op. You can make a copy of this frame to create a new Macro frame)"
        n209 = call <vilib>:"Add State(s) to Queue__jki_lib_state_machine.vi"("State(s) in (\"\")"=w513) -> ("States Out"=w512:string)  [unwired: 14 in]
      }
      frame "Macro: Initialize" {
        w514 = "Data: Initialize\nInitialize Core Data\nUI: Initialize\nUI: Front Panel State >> Open"  # Data: Initialize Initialize Core Data UI: Initialize UI: Front Panel State >> Open
        # "Initialization Macro\n(This is called once, when the VI starts)"
        n210 = call <vilib>:"Add State(s) to Queue__jki_lib_state_machine.vi"("State(s) in Front (\"\")"=w514, "State(s) in (\"\")"=w518) -> ("States Out"=w517:string)  [unwired: 13 in]
      }
      frame "Macro: Exit" {
        # "Exit Macro\n(This is called once, when the VI exits)"
        n211 = Unbundle By Name(w525) -> ("Core.Close Panel on Exit?"=w524:bool)
        n212 = Select(t="UI: Front Panel State >> Close", s=w524, f="") -> (s? t:f=w521:string)
        n213 = call <vilib>:"Add State(s) to Queue__jki_lib_state_machine.vi"("State(s) in (\"\")"=w521, "State(s) at Back (\"\")"="Data: Cleanup\nExit") -> ("States Out"=w519:string)  [unwired: 13 in]
        n214 = call <vilib>:"Add State(s) to Queue__jki_lib_state_machine.vi"("State(s) in Front (\"\")"=w519, "State(s) in (\"\")"=w528) -> ("States Out"=w527:string)  [unwired: 13 in]
      }
      frame "---------- New Category ----------" {
        # "Template Separator\n(You can make a copy of, or modify, this frame)"
        n215 = call <vilib>:"Add State(s) to Queue__jki_lib_state_machine.vi"("State(s) in (\"\")"=w532) -> ("States Out"=w531:string)  [unwired: 14 in]
      }
      frame "Update Averages" {
        n216 = local read "All Meter Data"() -> (w545:T10)
        n217 = Unbundle By Name(w539) -> ("Meter Data"=w540:T10)
        n218 = Unbundle By Name(w545) -> ("Meter Bank 1.Flow Rate (BTU/HR)"=w544:dbl, "Meter Bank 2.Flow Rate (BTU/HR)"=w543:dbl, "Meter Bank 3.Flow Rate (BTU/HR)"=w542:dbl)
        n219 = Bundle By Name(cluster=w540, "Meter Bank 1.Flow Rate (BTU/HR)"=w544, "Meter Bank 2.Flow Rate (BTU/HR)"=w543, "Meter Bank 3.Flow Rate (BTU/HR)"=w542) -> (w546:T10)
        n220 = call <vilib>:"Add State(s) to Queue__jki_lib_state_machine.vi"("State(s) in (\"\")"=w555) -> ("States Out"=w554:string)  [unwired: 14 in]
        n221 = call "RANGE Average Flow Rates.vi"("All Meter Data"=w546, "Error In"=w541, "Meter Number"=Range_Meter_Bank."Meter Bank 1") -> ("All Meter Data Out"=w551:T10, "Error Out"=w552:errorcluster)  [unwired: 15 in]
        n222 = call "RANGE Average Flow Rates.vi"("All Meter Data"=w551, "Error In"=w552, "Meter Number"=Range_Meter_Bank."Meter Bank 2") -> ("All Meter Data Out"=w550:T10, "Error Out"=w553:errorcluster)  [unwired: 15 in]
        n223 = call "RANGE Average Flow Rates.vi"("All Meter Data"=w550, "Error In"=w553, "Meter Number"=Range_Meter_Bank."Meter Bank 3") -> ("All Meter Data Out"=w537:T10, "Error Out"=w535:errorcluster)  [unwired: 15 in]
        "Average Updates" <- w537
        n224 = call "UTILITY Elapsed Time.vi"("error in (no error)"=w535) -> ("error out"=w534:errorcluster, "Main Loop Rate"=→"Main Loop Rate":dbl, "Elapsed Time"=w533:dbl)  [unwired: 6 in, 2 out]
        "Elapsed Time" <- w533
        n225 = Bundle By Name(cluster=w539, "Meter Data"=w537, "Elapsed Time DAQ"=w533) -> (w538:T20)
      }
      frame "ANSI Average Bank 1" {
        n226 = local read "All Meter Data"() -> (w567:T10)
        n227 = Unbundle By Name(w566) -> ("Bank 1 Counter"=w564:i32)
        n228 = call "RANGE ANSI Calculator.vi"("Meter Number"=Range_Meter_Bank."Meter Bank 1", "Error In"=w563, "All Meter Data"=w567, "Bank Counter"=w564) -> ("Error Out"=w562:errorcluster, "Count Down Timer"=w559:i32, "ANSI Average (BTU/HR)"=w557:dbl, "Bank Counter"=w558:i32, "Greater than 310 sec"=w561:bool)  [unwired: 3 in]
        "ANSI Average (BTU/hr)-Meter 1/2" <- w557
        n229 = case shown="True" w561 {
          frame False {
          }
          frame True {
            w570 = FALSE ("Start ANSI")
            n230 = local write "Start ANSI-S1"(w570) -> ()
            n231 = local write "Start ANSI"(w570) -> ()
          }
        }
        n232 = call "RANGE ANSI Message.vi"("Bank Counter"=w558, "Count Down Timer"=w559) -> ("ANSI Display 3"=→"ANSI Display 1" →"ANSI Display S1":string)  [unwired: 9 in]
        n233 = local write "ANSI Average (BTU/hr)"(w557) -> ()
        n234 = Bundle By Name(cluster=w566, "Bank 1 Counter"=w558) -> (w565:T20)
        n235 = call <vilib>:"Add State(s) to Queue__jki_lib_state_machine.vi"("State(s) in (\"\")"=w569) -> ("States Out"=w568:string)  [unwired: 14 in]
      }
      frame "ANSI Average Bank 2" {
        n236 = Unbundle By Name(w575) -> ("Bank 2 Counter"=w580:i32)
        n237 = local read "All Meter Data"() -> (w581:T10)
        n238 = call "RANGE ANSI Calculator.vi"("Meter Number"=Range_Meter_Bank."Meter Bank 2", "Error In"=w577, "All Meter Data"=w581, "Bank Counter"=w580) -> ("Error Out"=w576:errorcluster, "Count Down Timer"=w574:i32, "ANSI Average (BTU/HR)"=w572:dbl, "Bank Counter"=w573:i32, "Greater than 310 sec"=w582:bool)  [unwired: 3 in]
        "ANSI Average (BTU/hr)-Meter 3/4" <- w572
        n239 = case shown="True" w582 {
          frame False {
          }
          frame True {
            w585 = FALSE ("Start ANSI")
            n240 = local write "Start ANSI 2"(w585) -> ()
            n241 = local write "Start ANSI-S2"(w585) -> ()
          }
        }
        n242 = call "RANGE ANSI Message.vi"("Bank Counter"=w573, "Count Down Timer"=w574) -> ("ANSI Display 3"=→"ANSI Display 2" →"ANSI Display S2":string)  [unwired: 9 in]
        n243 = local write "ANSI Average (BTU/hr) 2"(w572) -> ()
        n244 = Bundle By Name(cluster=w575, "Bank 2 Counter"=w573) -> (w579:T20)
        n245 = call <vilib>:"Add State(s) to Queue__jki_lib_state_machine.vi"("State(s) in (\"\")"=w584) -> ("States Out"=w583:string)  [unwired: 14 in]
      }
      frame "ANSI Average Bank 3" {
        n246 = Unbundle By Name(w591) -> ("Bank 3 Counter"=w595:i32)
        n247 = local read "All Meter Data"() -> (w596:T10)
        n248 = call "RANGE ANSI Calculator.vi"("Meter Number"=Range_Meter_Bank."Meter Bank 3", "Error In"=w593, "All Meter Data"=w596, "Bank Counter"=w595) -> ("Error Out"=w590:errorcluster, "Count Down Timer"=w589:i32, "ANSI Average (BTU/HR)"=w587:dbl, "Bank Counter"=w588:i32, "Greater than 310 sec"=w597:bool)  [unwired: 3 in]
        "ANSI Average (BTU/hr)-Meter 5/6" <- w587
        n249 = case shown="True" w597 {
          frame False {
          }
          frame True {
            w600 = FALSE ("Start ANSI")
            n250 = local write "Start ANSI 3"(w600) -> ()
            n251 = local write "Start ANSI-S3"(w600) -> ()
          }
        }
        n252 = local write "ANSI Average (BTU/hr) 3"(w587) -> ()
        n253 = call "RANGE ANSI Message.vi"("Bank Counter"=w588, "Count Down Timer"=w589) -> ("ANSI Display 3"=→"ANSI Display 3" →"ANSI Display S3":string)  [unwired: 9 in]
        n254 = Bundle By Name(cluster=w591, "Bank 3 Counter"=w588) -> (w592:T20)
        n255 = call <vilib>:"Add State(s) to Queue__jki_lib_state_machine.vi"("State(s) in (\"\")"=w599) -> ("States Out"=w598:string)  [unwired: 14 in]
      }
      frame "Save Data" {
        n256 = call <vilib>:"Add State(s) to Queue__jki_lib_state_machine.vi"("State(s) in (\"\")"=w604) -> ("States Out"=w603:string)  [unwired: 14 in]
      }
      frame "Check Exit" {
        n257 = call "UTILITY Boolean Notifier.vi"("Status"=UTILITY_Notifier."Read", "name (unnamed)"="Exit") -> ("latest READ notification"=w606:bool)  [unwired: 8 in, 1 out]
        n258 = case shown="True" w606 {
          tunnel: ["" "Macro: Exit"] -> w605
          frame False {
          }
          frame True {
          }
        }
        n259 = call <vilib>:"Add State(s) to Queue__jki_lib_state_machine.vi"("State(s) in Front (\"\")"=w605, "State(s) in (\"\")"=w612) -> ("States Out"=w611:string)  [unwired: 13 in]
      }
    }
    n260 = case shown="False" "Debug" {
      tunnel: w53 -> [w65 w68]
      tunnel: [w65 w67] -> w52
      tunnel: w51 -> [_ w66]
      frame False {
      }
      frame True {
        n261 = Build Array (concatenate)(w68, w66) -> (w67:string[])
        "Debug Array" <- w67
      }
    }
    "ANSI Loop" <- w54
  }
  n262 = while {
    tunnel: w3 -> [w615]
    tunnel: [w615] -> w2
    i -> [w616]
    stop <- w623 stop-if-true
    n263 = local read "File Path"() -> (w617:path)
    n264 = Equal?(x=w617, y=path "") -> (x = y?=w618:bool)
    n265 = case shown="False" w618 {
      tunnel: w617 -> [w626 _]
      frame False {
        n266 = local read "All Meter Data"() -> (w628:T10)
        n267 = local read "Elapsed Time"() -> (w627:dbl)
        n268 = call "RANGE Write To File.vi"("Time"=w627, "All Meter Data"=w628, "File Path"=w626) -> ()  [unwired: 8 in, 1 out]
      }
      frame True {
      }
    }
    n269 = call "UTILITY Boolean Notifier.vi"("Status"=UTILITY_Notifier."Read", "name (unnamed)"="Exit") -> ("latest READ notification"=w623:bool)  [unwired: 8 in, 1 out]
    n270 = Multiply(x=T22 1000.0 ("y"), y="Scan Rate (Sec)") -> (x*y=w620:T22)
    n271 = Wait Until Next ms Multiple(millisecond multiple=w620) -> ()  [unwired: 1 out]
    "Save Loop" <- w616
  }
  n272 = while {
    tunnel: [w687] -> w15
    shift-right: [w704] -> _
    shift-left: w12 -> [w716]
    tunnel: w3 -> [w684]
    i -> [w674]
    stop <- w688 stop-if-true
    n273 = Bundle By Name(cluster=w716, "Threshold Voltage (NI DAQ)"="Rate Threshold (V)") -> (w715:T10)
    n274 = local read "Tot.Flow (SLPM Liters) Bank 1"() -> (w677:dbl)
    n275 = local read "Tot.Flow (SLPM Liters) Bank 2"() -> (w676:dbl)
    n276 = local read "Tot.Flow (SLPM Liters) Bank 3"() -> (w675:dbl)
    n277 = Bundle By Name(cluster=w715, "Meter Bank 1.Panel Data.Heating Value (BTU/ft³)"="HeatingValueS1", "Meter Bank 2.Panel Data.Heating Value (BTU/ft³)"="HeatingValueS2", "Meter Bank 3.Panel Data.Heating Value (BTU/ft³)"="HeatingValueS3") -> (w713:T10)
    n278 = call "RANGE GET Gas Data.vi"("DAQ Data In"=w713, "Tot.Flow (Liters) Bank 1"=w677, "Tot.Flow (Liters) Bank 2"=w676, "Tot.Flow (Liters) Bank 3"=w675, "Error In"=w684, "Meter Select 3"="Meter Select 3", "Meter Select 2"="Meter Select 2", "Meter Select 1"="Meter Select") -> ("DAQ Data Out"=w706:T10, "Error Out"=w702:errorcluster)  [unwired: 10 in]
    n279 = local read "Gas Mix Number Bank 1"() -> (w693:string)
    n280 = local read "Gas Mix Number Bank 2"() -> (w692:string)
    n281 = local read "Gas Mix Number Bank 3"() -> (w691:string)
    n282 = local read "Average Updates"() -> (w700:T10)
    n283 = call "RANGE General Data Processing.vi"("DAQ Data Out in"=w706, "Meter Select 3"="Meter Select 3", "Meter Select 2"="Meter Select 2", "Meter Select 1"="Meter Select", "error in (no error)"=w702) -> ("DAQ Data Out out"=w701:T10, "error out"=w703:errorcluster)  [unwired: 9 in]
    n284 = local read "ANSI 3"() -> (w681:bool)
    n285 = local read "ANSI 2"() -> (w682:bool)
    n286 = local read "ANSI 1"() -> (w683:bool)
    n287 = call "RANGE Update Averages.vi"("DAQ Data Out in"=w701, "Average Updates"=w700, "Error In"=w703, "Meter Bank 1.Start ANSI"=w683, "Gas Mix Number Bank 1"=w693, "Meter Bank 2.Start ANSI"=w682, "Gas Mix Number Bank 2"=w692, "Meter Bank 3.Start ANSI"=w681, "Gas Mix Number Bank 3"=w691) -> ("DAQ Data Out out"=w704:T10, "Error Out"=w686:errorcluster)  [unwired: 9 in]
    "All Meter Data" <- w704
    n288 = Unbundle By Name(w704) -> ("Meter Bank 1.Flow Rate (BTU/HR)"=w698:dbl, "Meter Bank 2.Flow Rate (BTU/HR)"=w697:dbl, "Meter Bank 3.Flow Rate (BTU/HR)"=w696:dbl, "Meter Bank 1.Panel Data"=→"Display Bank 1" →"Display S1":T6, "Meter Bank 2.Panel Data"=→"Display Bank 2" →"Display S2":T6, "Meter Bank 3.Panel Data"=→"Display Bank 3" →"Display S3":T6, "Meter Bank 1.Flow Rate (BTU/HR)"=w709:dbl, "Meter Bank 2.Flow Rate (BTU/HR)"=w708:dbl, "Meter Bank 3.Flow Rate (BTU/HR)"=w707:dbl, "Meter Bank 1.Meter ID"=w668:string, "Meter Bank 2.Meter ID"=w657:string, "Meter Bank 3.Meter ID"=w652:string, "Meter 1.Measurement Units"=w670:T12, "Meter 2.Measurement Units"=w669:T12, "Meter 3.Measurement Units"=w656:T12, "Meter 4.Measurement Units"=w655:T12, "Meter 5.Measurement Units"=w654:T12, "Meter 6.Measurement Units"=w653:T12)
    "Flow Rate S1" <- w698
    "Flow Rate S2" <- w697
    "Flow Rate S3" <- w696
    n289 = local write "Flow Rate"(w698) -> ()
    n290 = Bundle("Flow Rate (BTU/HR)"=w709) -> (→"DisplayChart" →"Station 1 Chart":cluster{"Flow Rate (BTU/HR)":dbl})  [unwired: 1 in]
    n291 = Bundle("Flow Rate (BTU/HR)"=w708) -> (→"DisplayChart 2" →"Station 2 Chart":cluster{"Flow Rate (BTU/HR)":dbl})  [unwired: 1 in]
    n292 = Bundle("Flow Rate (BTU/HR)"=w707) -> (→"DisplayChart 3" →"Station 3 Chart":cluster{"Flow Rate (BTU/HR)":dbl})  [unwired: 1 in]
    n293 = while {
      tunnel: w668 -> [w796]
      shift-right: [w795] -> _
      shift-left: _ -> [w804]
      tunnel: w657 -> [w794]
      shift-right: [w793] -> _
      shift-left: _ -> [w803]
      tunnel: w652 -> [w797]
      shift-right: [w792] -> _
      shift-left: _ -> [w802]
      stop <- TRUE stop-if-true
      # "Auto Switch Tab FGV"
      n294 = Not Equal?(x=w804, y=w796) -> (x != y?=w800:bool)
      n295 = Not Equal?(x=w803, y=w794) -> (x != y?=w799:bool)
      n296 = Not Equal?(x=w802, y=w797) -> (x != y?=w798:bool)
      n297 = Compound Arithmetic op=OR(w800, w799, w798) -> (w801:bool)
      n298 = case shown="True" w801 {
        tunnel: w796 -> [w806 w817]
        tunnel: w800 -> [_ w816]
        tunnel: w799 -> [_ w815]
        tunnel: w794 -> [w808 w814]
        tunnel: w798 -> [_ w813]
        tunnel: w797 -> [w807 w812]
        tunnel: [w806 w811] -> w795
        tunnel: [w808 w810] -> w793
        tunnel: [w807 w809] -> w792
        frame False {
        }
        frame True {
          n299 = case shown="True" w816 {
            tunnel: w817 -> [w832 w835]
            tunnel: [w832 "" ("Meter ID")] -> w811
            frame False {
            }
            frame True {
              n300 = case shown="\"B\"" w835 {
                selector: w835 -> [w836 _ _]
                tunnel: [w836 "1" "2"] -> w834
                frame Default {
                }
                frame "A" {
                }
                frame "B" {
                }
              }
              n301 = property on="Meter 1/2" class="Str"("Val(Sgnl)"=w834) -> ()  [unwired: 2 in, 2 out]
            }
          }
          n302 = case shown="True" w815 {
            tunnel: w814 -> [w825 w828]
            tunnel: [w825 "" ("Meter ID")] -> w810
            frame False {
            }
            frame True {
              n303 = case shown="\"D\"" w828 {
                selector: w828 -> [w829 _ _]
                tunnel: [w829 "3" "4"] -> w827
                frame Default {
                }
                frame "C" {
                }
                frame "D" {
                }
              }
              n304 = property on="Meter 3/4" class="Str"("Val(Sgnl)"=w827) -> ()  [unwired: 2 in, 2 out]
            }
          }
          n305 = case shown="True" w813 {
            tunnel: w812 -> [w818 w821]
            tunnel: [w818 "" ("Meter ID")] -> w809
            frame False {
            }
            frame True {
              n306 = case shown="Default" w821 {
                selector: w821 -> [w822 _ _]
                tunnel: [w822 "5" "6"] -> w820
                frame Default {
                }
                frame "E" {
                }
                frame "F" {
                }
              }
              n307 = property on="Meter 5/6" class="Str"("Val(Sgnl)"=w820) -> ()  [unwired: 2 in, 2 out]
            }
          }
        }
      }
    }
    n308 = call <vilib>:"Clear Errors.vi"("error in (no error)"=w686) -> ("error out"=w685:errorcluster)  [unwired: 5 in, 1 out]
    n309 = local write "Flow Rate 2"(w697) -> ()
    n310 = local write "Flow Rate 3"(w696) -> ()
    n311 = case shown="\"C\"" w657 {
      tunnel: w656 -> [w743 _ _]
      tunnel: w655 -> [_ w755 _]
      tunnel: [w753 w765 w766] -> w651
      tunnel: [w752 w764 w766] -> w650
      tunnel: [w751 w763 w766] -> w649
      tunnel: [w750 w762 w766] -> w648
      tunnel: [w749 w761 w766] -> w647
      tunnel: [w748 w760 w766] -> w646
      tunnel: [w747 w759 w766] -> w645
      tunnel: [w746 w758 w766] -> w644
      tunnel: [w745 w757 w766] -> w643
      tunnel: [w744 w756 w766] -> w642
      tunnel: [w742 w754 w766] -> w630
      frame "C" {
        n312 = Unbundle By Name(w743) -> ("Abs. Pressure"=w748:string, "Temperature"=w747:string, "Volume"=w746:string, "Mass"=w745:string, "Totalizer"=w744:string, "Software Version"=w742:string)
        n313 = Unbundle By Name(w743) -> ("Abs. Pressure"=w753:string, "Temperature"=w752:string, "Volume"=w751:string, "Mass"=w750:string, "Totalizer"=w749:string)
      }
      frame "D" {
        n314 = Unbundle By Name(w755) -> ("Abs. Pressure"=w760:string, "Temperature"=w759:string, "Volume"=w758:string, "Mass"=w757:string, "Totalizer"=w756:string, "Software Version"=w754:string)
        n315 = Unbundle By Name(w755) -> ("Abs. Pressure"=w765:string, "Temperature"=w764:string, "Volume"=w763:string, "Mass"=w762:string, "Totalizer"=w761:string)
      }
      frame Default {
        w766 = "" ("Abs. Pressure")
      }
    }
    "Bank 2 Mass Flow" <- w648
    "Bank 2 Vol Flow" <- w649
    "Bank 2 Tot. Flow" <- w647
    "Bank 2 Gas Temp" <- w650
    "Bank 2 Gas Pres" <- w651
    "Bank 2 Mass Flow 2" <- w643
    "Bank 2 Vol Flow 3" <- w644
    "Bank 2 Tot. Flow 3" <- w642
    "Bank 2 Gas Temp 3" <- w645
    "Bank 2 Gas Pres 3" <- w646
    "Meter Software 3/4" <- w630
    n316 = case shown="\"E\"" w652 {
      tunnel: w654 -> [w718 _ _]
      tunnel: w653 -> [_ w730 _]
      tunnel: [w728 w740 w741] -> w641
      tunnel: [w727 w739 w741] -> w640
      tunnel: [w726 w738 w741] -> w639
      tunnel: [w725 w737 w741] -> w638
      tunnel: [w724 w736 w741] -> w637
      tunnel: [w723 w735 w741] -> w636
      tunnel: [w722 w734 w741] -> w635
      tunnel: [w721 w733 w741] -> w634
      tunnel: [w720 w732 w741] -> w633
      tunnel: [w719 w731 w741] -> w632
      tunnel: [w717 w729 w741] -> w629
      frame "E" {
        n317 = Unbundle By Name(w718) -> ("Abs. Pressure"=w723:string, "Temperature"=w722:string, "Volume"=w721:string, "Mass"=w720:string, "Totalizer"=w719:string, "Software Version"=w717:string)
        n318 = Unbundle By Name(w718) -> ("Abs. Pressure"=w728:string, "Temperature"=w727:string, "Volume"=w726:string, "Mass"=w725:string, "Totalizer"=w724:string)
      }
      frame "F" {
        n319 = Unbundle By Name(w730) -> ("Abs. Pressure"=w735:string, "Temperature"=w734:string, "Volume"=w733:string, "Mass"=w732:string, "Totalizer"=w731:string, "Software Version"=w729:string)
        n320 = Unbundle By Name(w730) -> ("Abs. Pressure"=w740:string, "Temperature"=w739:string, "Volume"=w738:string, "Mass"=w737:string, "Totalizer"=w736:string)
      }
      frame Default {
        w741 = "" ("Abs. Pressure")
      }
    }
    "Bank 3 Mass Flow" <- w638
    "Bank 3 Vol Flow" <- w639
    "Bank 3 Tot. Flow" <- w637
    "Bank 3 Gas Temp" <- w640
    "Bank 3 Gas Pres" <- w641
    "Bank 3 Mass Flow" <- w633
    "Bank 3 Vol Flow" <- w634
    "Bank 3 Gas Temp" <- w635
    "Bank 3 Gas Pres" <- w636
    "Bank 3 Tot. Flow" <- w632
    "Meter Software 5/6" <- w629
    n321 = case shown="Default" w668 {
      tunnel: w670 -> [w768 _ _]
      tunnel: w669 -> [_ w780 _]
      tunnel: [w778 w790 w791] -> w667
      tunnel: [w777 w789 w791] -> w666
      tunnel: [w776 w788 w791] -> w665
      tunnel: [w775 w787 w791] -> w664
      tunnel: [w774 w786 w791] -> w663
      tunnel: [w773 w785 w791] -> w662
      tunnel: [w772 w784 w791] -> w661
      tunnel: [w771 w783 w791] -> w660
      tunnel: [w770 w782 w791] -> w659
      tunnel: [w769 w781 w791] -> w658
      tunnel: [w767 w779 w791] -> w631
      frame "A" {
        n322 = Unbundle By Name(w768) -> ("Abs. Pressure"=w773:string, "Temperature"=w772:string, "Volume"=w771:string, "Mass"=w770:string, "Totalizer"=w769:string, "Software Version"=w767:string)
        n323 = Unbundle By Name(w768) -> ("Abs. Pressure"=w778:string, "Temperature"=w777:string, "Volume"=w776:string, "Mass"=w775:string, "Totalizer"=w774:string)
      }
      frame "B" {
        n324 = Unbundle By Name(w780) -> ("Abs. Pressure"=w785:string, "Temperature"=w784:string, "Volume"=w783:string, "Mass"=w782:string, "Totalizer"=w781:string, "Software Version"=w779:string)
        n325 = Unbundle By Name(w780) -> ("Abs. Pressure"=w790:string, "Temperature"=w789:string, "Volume"=w788:string, "Mass"=w787:string, "Totalizer"=w786:string)
      }
      frame Default {
        w791 = "" ("Abs. Pressure")
      }
    }
    "Bank 1 Mass Flow" <- w664
    "Bank 1 Vol Flow" <- w665
    "Bank 1 Tot. Flow" <- w663
    "Bank 1 Gas Temp" <- w666
    "Bank 1 Gas Pres" <- w667
    "Bank 1 Mass Flow" <- w659
    "Bank 1 Vol Flow" <- w660
    "Bank 1 Gas Temp" <- w661
    "Bank 1 Gas Pres" <- w662
    "Bank 1 Tot. Flow" <- w658
    "Meter Software 1/2" <- w631
    n326 = call "UTILITY Boolean Notifier.vi"("Status"=UTILITY_Notifier."Read", "error in (no error)"=w685, "name (unnamed)"="Exit") -> ("error out"=w687:errorcluster, "latest READ notification"=w688:bool)  [unwired: 7 in]
    n327 = Wait Until Next ms Multiple(millisecond multiple=u32 250) -> ()  [unwired: 1 out]
    "Main Control Loop" <- w674
  }
  n328 = while {
    tunnel: w3 -> [w839]
    tunnel: [w839] -> w1
    i -> [w840]
    stop <- w841 stop-if-true
    n329 = event shown="[3] \"Meter 5/6\": Value Change" {
      selector: _ -> [_ _ _ _]
      dyn-events: _ -> [_ _ _ _]
      timeout: _ -> [_ _ _ _]
      event Timeout {
        n330 = event-data() -> ()  [unwired: 1 in, 3 out]
      }
      event "Meter 1/2": Value Change {
        n331 = event-data() -> ("NewVal"=w844:string)  [unwired: 1 in, 5 out]
        n332 = local read "Meter Select"() -> (w845:T3)
        n333 = case shown="\"Auto\"" w845 {
          tunnel: w844 -> [_ w852]
          frame Default {
          }
          frame "Auto" {
            n334 = local read "All Meter Data"() -> (w851:T10)
            n335 = Unbundle By Name(w851) -> ("Use Auto Switching"=w847:bool, "Meter Bank 1.Panel Data.Mass Flow"=w849:dbl)
            n336 = Greater Than 0?(x=w849) -> (x > 0?=w848:bool)
            n337 = And(x=w847, y=w848) -> (x .and. y?=w846:bool)
            n338 = case shown="True" w846 {
              tunnel: [TRUE w854] -> w850
              frame False {
              }
              frame True {
                n339 = local read "Tab Control 2"() -> (w858:T1)
                n340 = Equal?(x=w858, y=T1."All Stations" ("Tab Control 2")) -> (x = y?=w856:bool)
                n341 = Equal?(x=w858, y=T1."Custom Gases") -> (x = y?=w855:bool)
                n342 = Compound Arithmetic op=OR(w856, w855) -> (w854:bool)
              }
            }
            n343 = case shown="False" w850 {
              tunnel: w852 -> [w860 _]
              frame False {
                n344 = case shown="\"1\", \"2\"" w860 {
                  frame Default {
                  }
                  frame "1", "2" {
                    n345 = local write "Tab Control 2"(T1."Meter 1 & 2" ("Tab Control 2")) -> ()
                  }
                }
              }
              frame True {
              }
            }
          }
        }
      }
      event "Meter 3/4": Value Change {
        n346 = event-data() -> ("NewVal"=w863:string)  [unwired: 1 in, 5 out]
        n347 = local read "Meter Select 2"() -> (w862:T4)
        n348 = case shown="\"Auto\"" w862 {
          tunnel: w863 -> [_ w870]
          frame Default {
          }
          frame "Auto" {
            n349 = local read "All Meter Data"() -> (w865:T10)
            n350 = Unbundle By Name(w865) -> ("Use Auto Switching"=w866:bool, "Meter Bank 2.Panel Data.Mass Flow"=w868:dbl)
            n351 = Greater Than 0?(x=w868) -> (x > 0?=w867:bool)
            n352 = And(x=w866, y=w867) -> (x .and. y?=w864:bool)
            n353 = case shown="True" w864 {
              tunnel: [TRUE w872] -> w869
              frame False {
              }
              frame True {
                n354 = local read "Tab Control 2"() -> (w876:T1)
                n355 = Equal?(x=w876, y=T1."All Stations" ("Tab Control 2")) -> (x = y?=w874:bool)
                n356 = Equal?(x=w876, y=T1."Custom Gases") -> (x = y?=w873:bool)
                n357 = Compound Arithmetic op=OR(w874, w873) -> (w872:bool)
              }
            }
            n358 = case shown="False" w869 {
              tunnel: w870 -> [w878 _]
              frame False {
                n359 = case shown="\"3\", \"4\"" w878 {
                  frame Default {
                  }
                  frame "3", "4" {
                    n360 = local write "Tab Control 2"(T1."Meter 3 & 4" ("Tab Control 2")) -> ()
                  }
                }
              }
              frame True {
              }
            }
          }
        }
      }
      event "Meter 5/6": Value Change {
        n361 = event-data() -> ("NewVal"=w881:string)  [unwired: 1 in, 5 out]
        n362 = local read "Meter Select 3"() -> (w880:T5)
        n363 = case shown="Default" w880 {
          tunnel: w881 -> [_ w888]
          frame Default {
          }
          frame "Auto" {
            n364 = local read "All Meter Data"() -> (w883:T10)
            n365 = Unbundle By Name(w883) -> ("Use Auto Switching"=w884:bool, "Meter Bank 3.Panel Data.Mass Flow"=w886:dbl)
            n366 = Greater Than 0?(x=w886) -> (x > 0?=w885:bool)
            n367 = And(x=w884, y=w885) -> (x .and. y?=w882:bool)
            n368 = case shown="True" w882 {
              tunnel: [TRUE w890] -> w887
              frame False {
              }
              frame True {
                n369 = local read "Tab Control 2"() -> (w894:T1)
                n370 = Equal?(x=w894, y=T1."All Stations" ("Tab Control 2")) -> (x = y?=w892:bool)
                n371 = Equal?(x=w894, y=T1."Custom Gases") -> (x = y?=w891:bool)
                n372 = Compound Arithmetic op=OR(w892, w891) -> (w890:bool)
              }
            }
            n373 = case shown="False" w887 {
              tunnel: w888 -> [w896 _]
              frame False {
                n374 = case shown="\"5\", \"6\"" w896 {
                  frame Default {
                  }
                  frame "5", "6" {
                    n375 = local write "Tab Control 2"(T1."Meter 5 & 6" ("Tab Control 2")) -> ()
                  }
                }
              }
              frame True {
              }
            }
          }
        }
      }
    }
    n376 = call "UTILITY Boolean Notifier.vi"("Status"=UTILITY_Notifier."Read", "name (unnamed)"="Exit") -> ("latest READ notification"=w841:bool)  [unwired: 8 in, 1 out]
    "Event Loop" <- w840
  }
  n377 = while {
    shift-right: [w912] -> _
    shift-left: w13 -> [w915]
    shift-right: [w911] -> _
    shift-left: w13 -> [w914]
    shift-right: [w910] -> _
    shift-left: w13 -> [w913]
    tunnel: w3 -> [w917]
    tunnel: [w898] -> w5
    i -> [w900]
    stop <- w901 stop-if-true
    # "Integrate SLPM becasue it accounts for STP"
    n378 = local read "All Meter Data"() -> (w918:T10)
    n379 = Unbundle By Name(w918) -> ("Meter Bank 1.Panel Data.Mass Flow"=w906:dbl, "Meter Bank 2.Panel Data.Mass Flow"=w905:dbl, "Meter Bank 3.Panel Data.Mass Flow"=w904:dbl)
    n380 = call "FMA1600A Get Bank Total Flow.vi"("Integral Array Input 1"=w915, "Integral Array Input 2"=w914, "Integral Array Input -3"=w913, "Min to Sec Convert (Total Flow)"="Min to Sec Convert (Total Flow)", "error in (no error)"=w917, "LPM (Vol. Flow) 1"=w906, "LPM (Vol. Flow) 2"=w905, "LPM (Vol. Flow) 3"=w904) -> ("Tot.Flow (Liters) Bank 1"=→"Tot.Flow (SLPM Liters) Bank 1":dbl, "Tot.Flow (Liters) Bank 2"=→"Tot.Flow (SLPM Liters) Bank 2":dbl, "Tot.Flow (Liters) Bank 3"=→"Tot.Flow (SLPM Liters) Bank 3":dbl, "Integral Array Output 1"=w912:dbl[], "Integral Array Output 2"=w911:dbl[], "Integral Array Output-3"=w910:dbl[], "error out"=w899:errorcluster)  [unwired: 1 in]
    n381 = call "UTILITY Boolean Notifier.vi"("Status"=UTILITY_Notifier."Read", "error in (no error)"=w899, "name (unnamed)"="Exit") -> ("error out"=w898:errorcluster, "latest READ notification"=w901:bool)  [unwired: 7 in]
    "Gas Total Loop" <- w900
  }
  n382 = Merge Errors(w2, w1, w5, w14, w15) -> (w7:errorcluster)
  n383 = call <vilib>:"Clear Errors.vi"("error in (no error)"=w7) -> ("error out"=w6:errorcluster)  [unwired: 5 in, 1 out]
  n384 = call "UTILITY Boolean Notifier.vi"("Status"=UTILITY_Notifier."Release Ref", "error in (no error)"=w6, "Set Status"=FALSE, "name (unnamed)"="Exit") -> ("error out"=→"Error Out":errorcluster)  [unwired: 6 in, 1 out]
